vi "Main HMI.vi"() -> ()   [LabVIEW 2020]
uses:
  Control/State - Main HMI.ctl
  Control/Page List Configuration.ctl
  <vilib>/Utility/miscctls.llb/LVRectTypeDef.ctl
  Control/Setup - Sequence Data.ctl
  <vilib>/Utility/miscctls.llb/LVPointTypeDef.ctl
  <vilib>/Utility/miscctls.llb/LVPositionTypeDef.ctl
  Control/State - FGV.ctl
  <vilib>/picture/picture.llb/imagedata.ctl
  Control/Header - Page.ctl
  <vilib>/Utility/miscctls.llb/LVBoundsTypeDef.ctl
  Control/State - eFGV.ctl
  Control/Header - User Management.ctl
  Control/Section.ctl
  <vilib>/Platform/browser.llb/Open URL in Default Browser (string).vi
panel:
  out "Project Name":string
  out "Version":string="v1.0"
  in  "Developer":bool
  out "Logo":picture
  in  "Acquire":bool
  out "Log Time":dbl format="%<%H:%M:%S>t"
  in  "Log":bool
  in  "Left":bool caption="1"
  in  "Page":T1(radio)=enum."2"
  in  "Right":bool caption="11"
  in  "Screenshot":bool
  in  "Info":bool
  in  "Alarm Event":bool
  in  "Logout":bool
  in  "Close":bool
  out "Disable":bool
  in  "Error in":errorcluster
  out "Error out":errorcluster
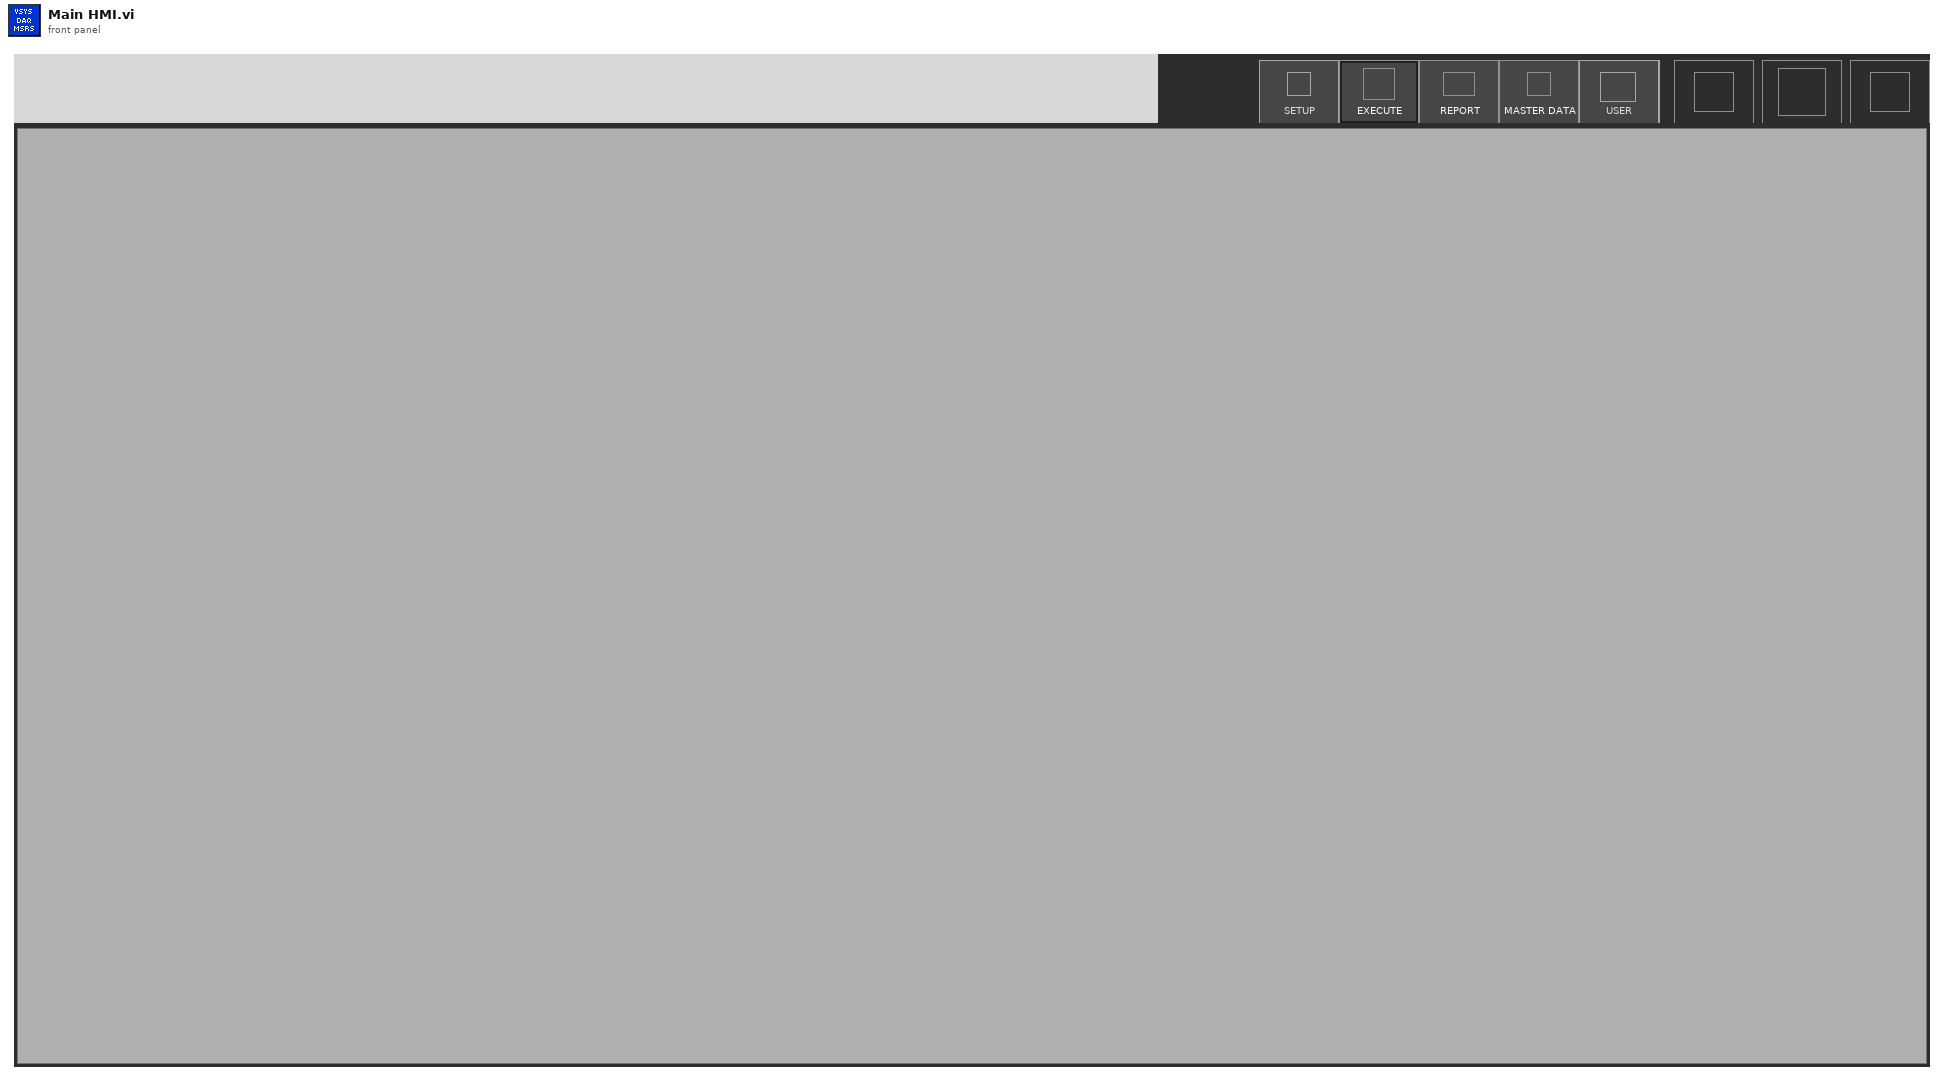
[diagram p1: front panel]
types:
  T1 = enum32{"1", "2", "3", "4", "5", "6", "7", "8", "9", "10", "11", "12", "13", "14", "15"}
  T2 = typedef "Page List Configuration.ctl" = cluster{"HMI Configuration":cluster{"EXE Name":string, "Project Name":string, "Max Page No":i32, "HMI State":enum32{"Invalid", "Standard", "Closed", "Hidden", "Minimized", "Maximized"}, "Version":enum16{"Demo", "User"}, "Check License":bool, "Font Size":u32, "Res: Height":i16, "Res: Width":i16, "License Level":enum16{"Level 1", "Level 2", "Level 3", "Level 4", "Level 5"}, "License Type":enum16{"Free", "Trial", "Subscription", "Perpetual"}}, "All HMI Module":string[], "Default HMI Module":string[], "Page Module":string[], "Page List: Level 1":string[], "Page List: Level 2":string[], "Page List: Level 3":string[], "All RT Module":string[], "Default RT Module":string[], "Acquire Enable Page":string[], "Log Enable Page":string[], "Run Page":string[], "Kill Page":string[], "Button":cluster{"Text":string[], "Tip Strip":string[]}}
  T3 = typedef "LVRectTypeDef.ctl" = cluster{"Left":i16, "Top":i16, "Right":i16, "Bottom":i16}
  T4 = typedef "Setup - Sequence Data.ctl" = cluster{"Seq.Select":bool, "Seq.Status":u32, "Seq.Run":bool, "Seq.TestSequence":string, "Seq.No":string, "Seq.ReqID":string, "Seq.TestReq":string, "Seq.Variance":string, "Seq.TestProcedure":string, "Seq.Section":string, "Seq.TestBunker":string, "Seq.TestMedia":string, "Seq.TestPressure":string, "Seq.Cycle":string, "Seq.HoldingTime":string, "Seq.ChartScale":string, "Seq.BDIndicator":string, "Seq.ActuatorPressure":string, "Seq.MaxBDPressure":string}
  T5 = cluster{"Config":T2, "Module":cluster{"Run Module":string[], "Kill Module":string[], "Page Module":string[], "Enable Page":string[]}, "Page Name":string, "T_Out":i32, "Time":timestamp, "Acquire":bool, "Log":bool, "Login":bool, "Discover":bool, "Button Ref":refnum<vi>[], "Direction":string, "Page Size":i32, "Content Area Rect":T3, "Page Size (Hidden)":i32, "Force Logout?":bool, "Update Button":bool, "Sequence Data":T4[], "Event Ref":refnum<event-registration>}
  T6 = typedef "State - Main HMI.ctl" = enum16{"Init", "Init Logo & Name", "Init Size", "Init Page", "Init Button Page", "Init Splitter", "Register Events", "Init Module", "Run Module", "Kill Module", "Change Page", "Update Button Page", "Close Splash Screen", "Idle", "Screenshot", "Developer Mode", "Info", "Move Button Page", "Acquire Event", "Log Event", "Logout", "Check for Exit", "Close"}
  T7 = enum32{"invalid app kind", "Development System", "Run Time System", "Student Edition", "Embedded LabVIEW", "Evaluation", "Custom"}
  T8 = typedef "LVPositionTypeDef.ctl" = cluster{"Left":i32, "Top":i32}
  T9 = typedef "State - FGV.ctl" = enum16{"Write", "Read"}
  T10 = typedef "imagedata.ctl" = cluster{"image type":i32, "image depth":i32, "image":u8[], "mask":u8[], "colors":u32[], "Rectangle":cluster{"left":i16, "top":i16, "right":i16, "bottom":i16}}
  T11 = enum16{"Init", "Init Module", "Run Module", "Kill Module", "Change Page", "Exit"}
  T12 = typedef "Header - Page.ctl" = enum16{"P1 Main", "P2", "P3 Analysis", "P4 Prediction", "P5 User"}
  T13 = enum8{"Enabled", "Disabled", "Disabled and Grayed Out"}
  T14 = typedef "LVBoundsTypeDef.ctl" = cluster{"Width":u32, "Height":u32}
  T15 = typedef "Header - User Management.ctl" = enum16{"Name", "Staff ID", "Username", "Password", "Access Level", "Status", "Access Page"}
  T16 = enum32{"Invalid", "Standard", "Closed", "Hidden", "Minimized", "Maximized"}
  T17 = typedef "Section.ctl" = enum16{"Software Setup", "Config", "Setup", "Network Stream", "MQTT Client", "Setting", "Sample Interval", "Calibration", "Pre-Ranging", "Overrun", "Static", "Filter", "Properties", "Alarm", "Device", "Logging"}
  T18 = typedef "LVPointTypeDef.ctl" = cluster{"Horizontal":i16, "Vertical":i16}
  T19 = typedef "State - eFGV.ctl" = enum16{"Init", "Read", "Write", "Exit"}
  T20 = typedef "License File Parameter.ctl" = cluster{"Expired Time":string, "Computer ID":string, "Product Name":string, "Period":i16, "Activated Time":string, "License Level":enum16{"Level 1", "Level 2", "Level 3", "Level 4", "Level 5"}, "License Type":enum16{"Free", "Trial", "Subscription", "Perpetual"}, "Log Time":string}
  T21 = enum16{"Free", "Trial", "Subscription", "Perpetual"}
  T22 = cluster{"Page Name":string, "All Module":string[], "Default Run Module":string[], "Page Module":string[]}
  T23 = enum16{"Level 1", "Level 2", "Level 3", "Level 4", "Level 5"}
  T24 = enum16{"Pre-Ranging", "Overrun", "Static", "Analysis", "Prediction"}
  T25 = enum32{"Bad", "Idle", "Run top level", "Running"}
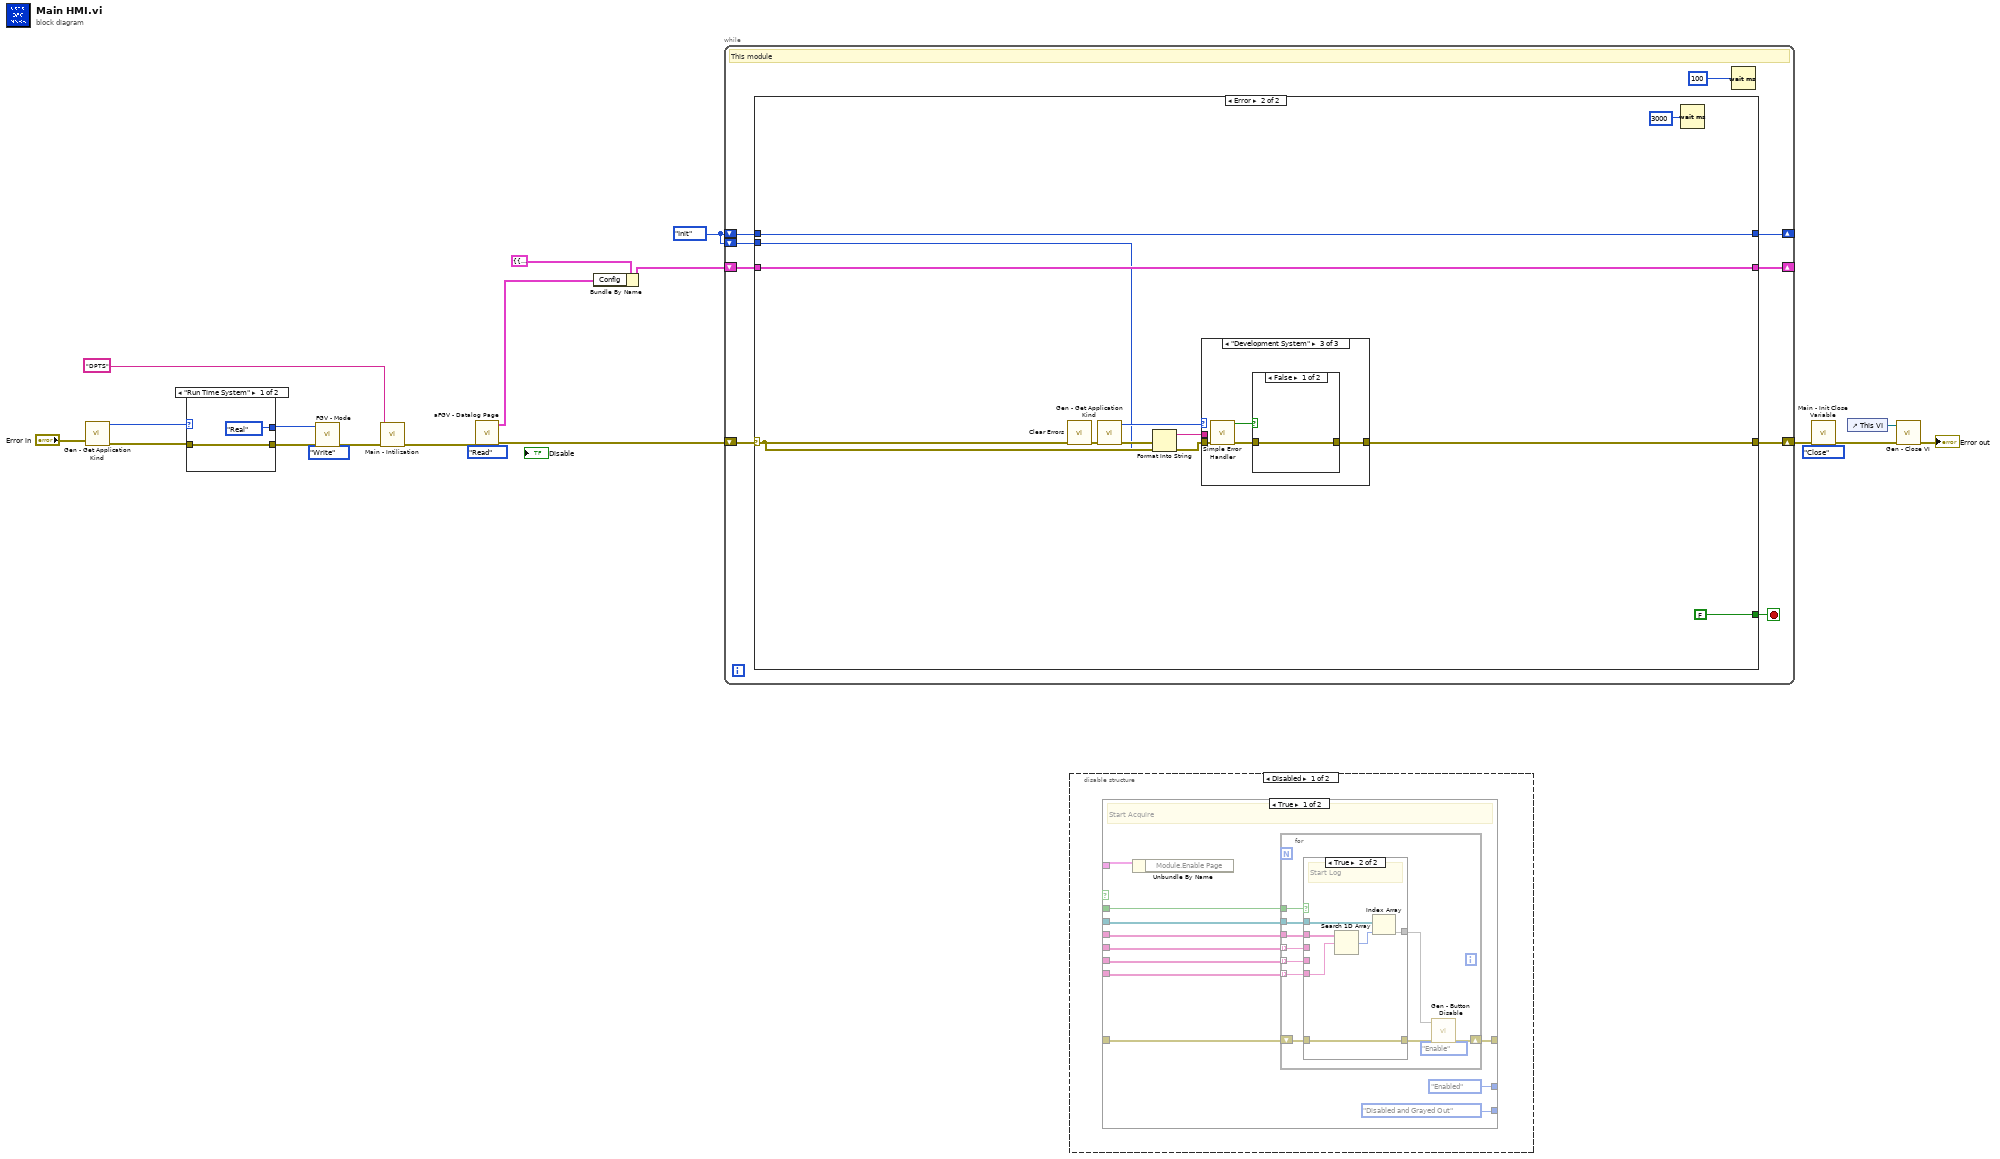
[diagram p0: block diagram]
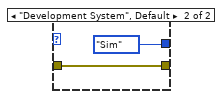
[diagram p2: hidden frame]
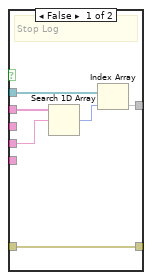
[diagram p3: hidden frame]
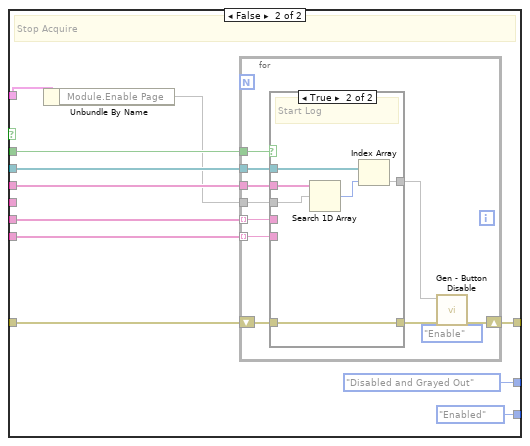
[diagram p4: hidden frame]
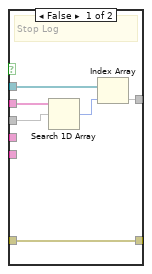
[diagram p5: hidden frame]
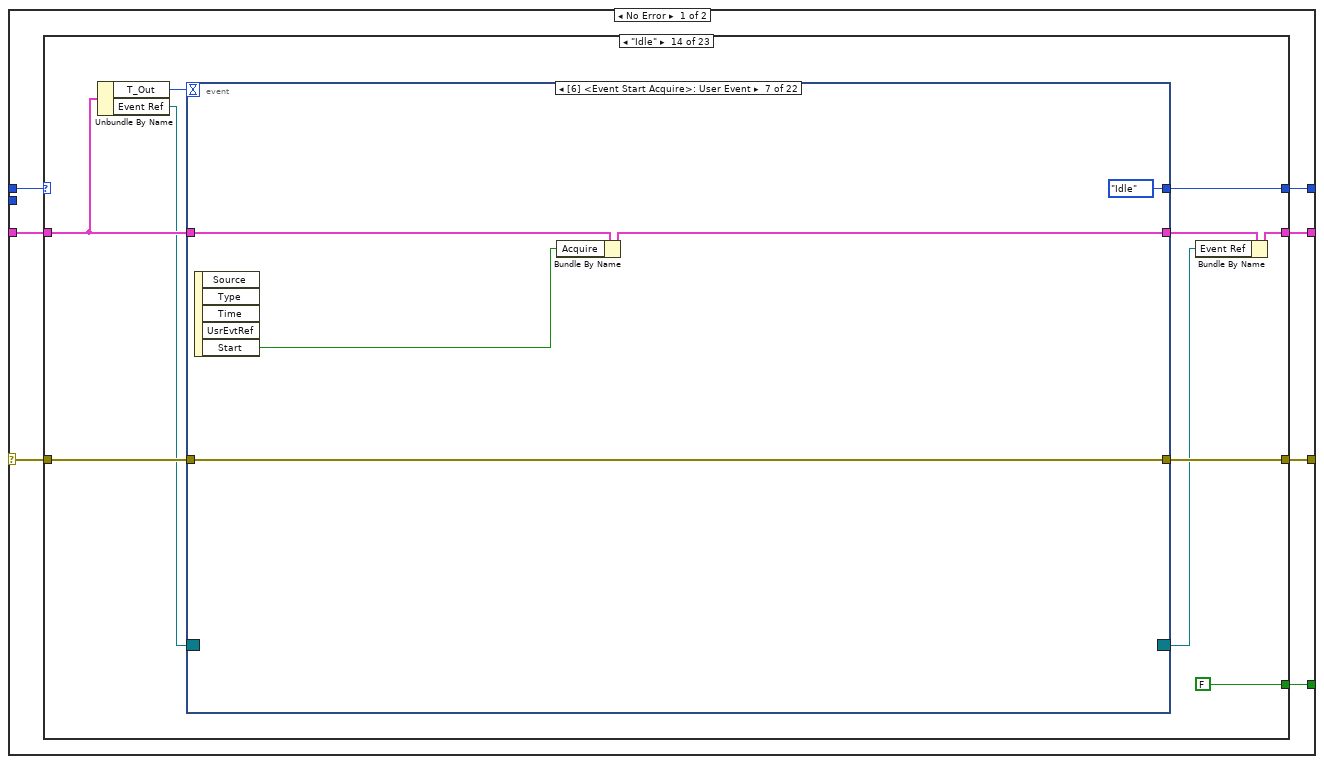
[diagram p7: hidden frame]
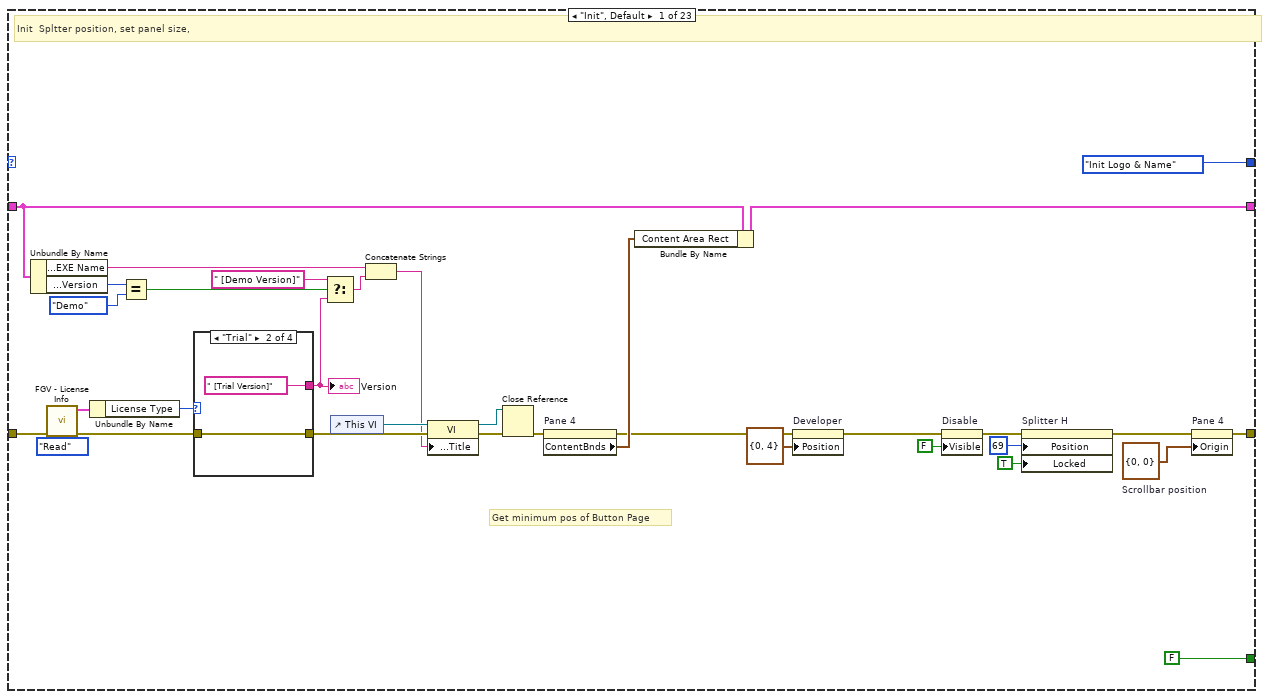
[diagram p8: hidden frame]
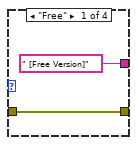
[diagram p9: hidden frame]
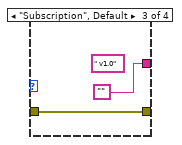
[diagram p10: hidden frame]
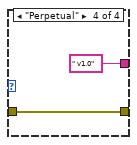
[diagram p11: hidden frame]
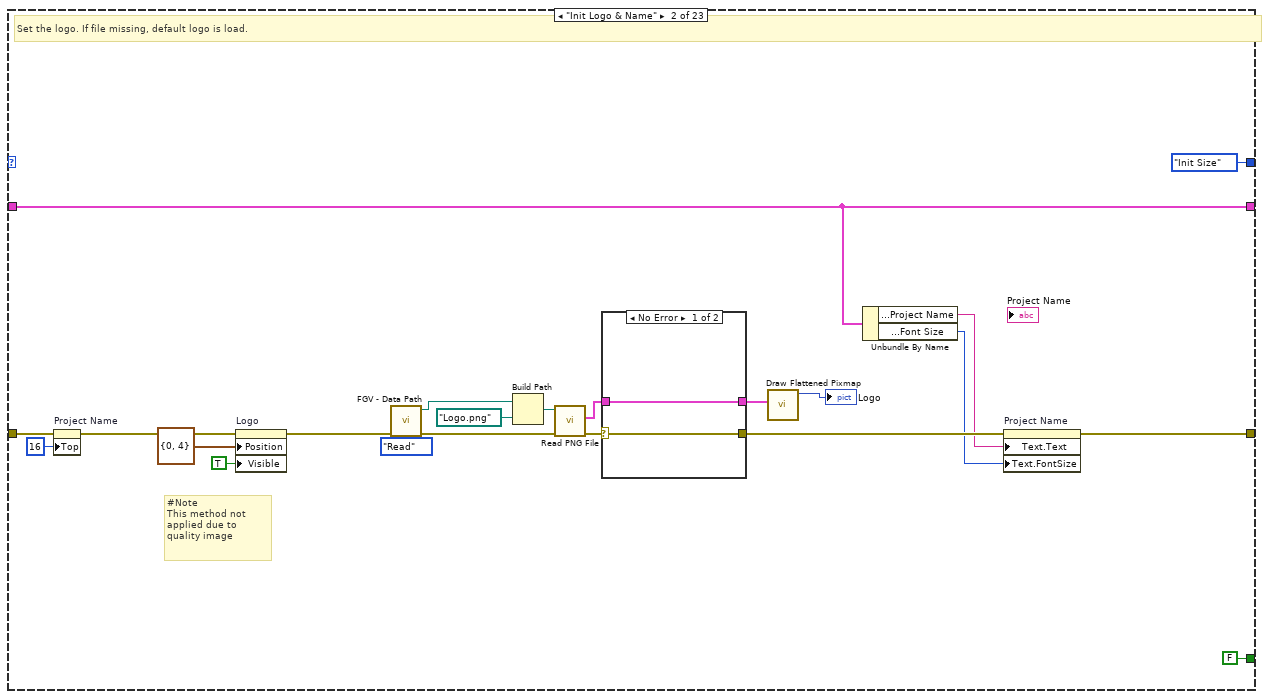
[diagram p12: hidden frame]
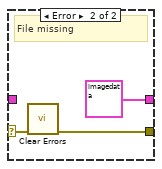
[diagram p13: hidden frame]
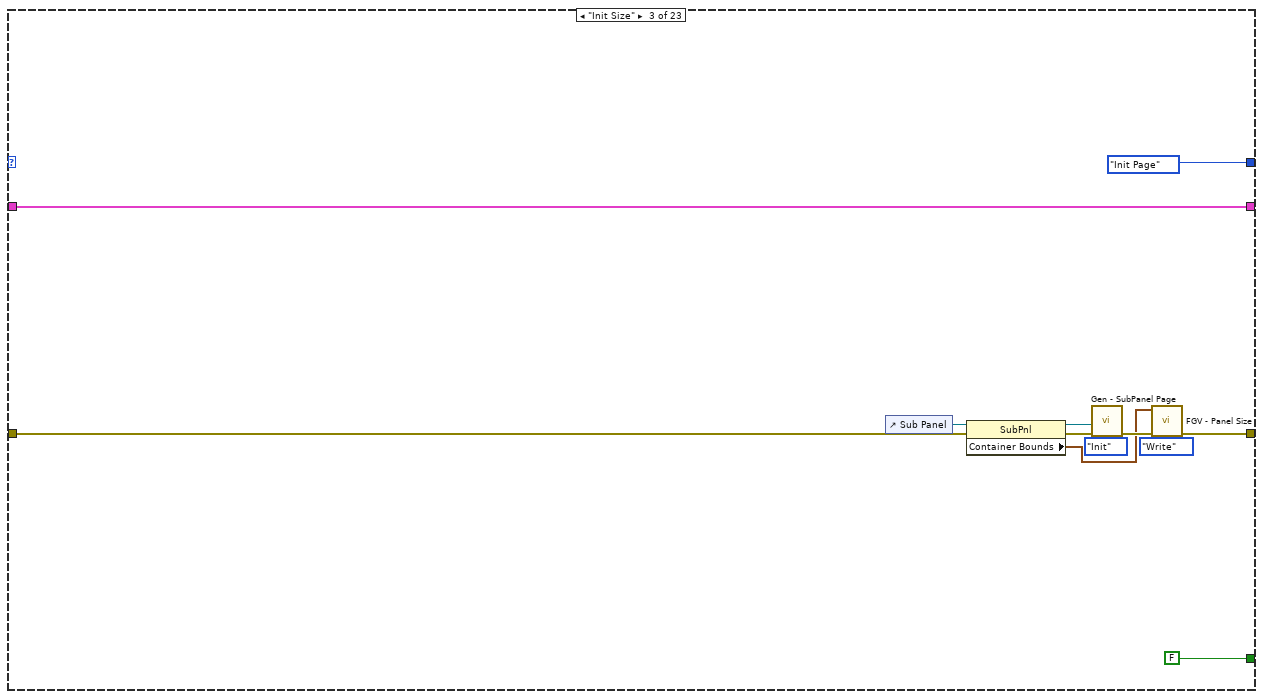
[diagram p14: hidden frame]
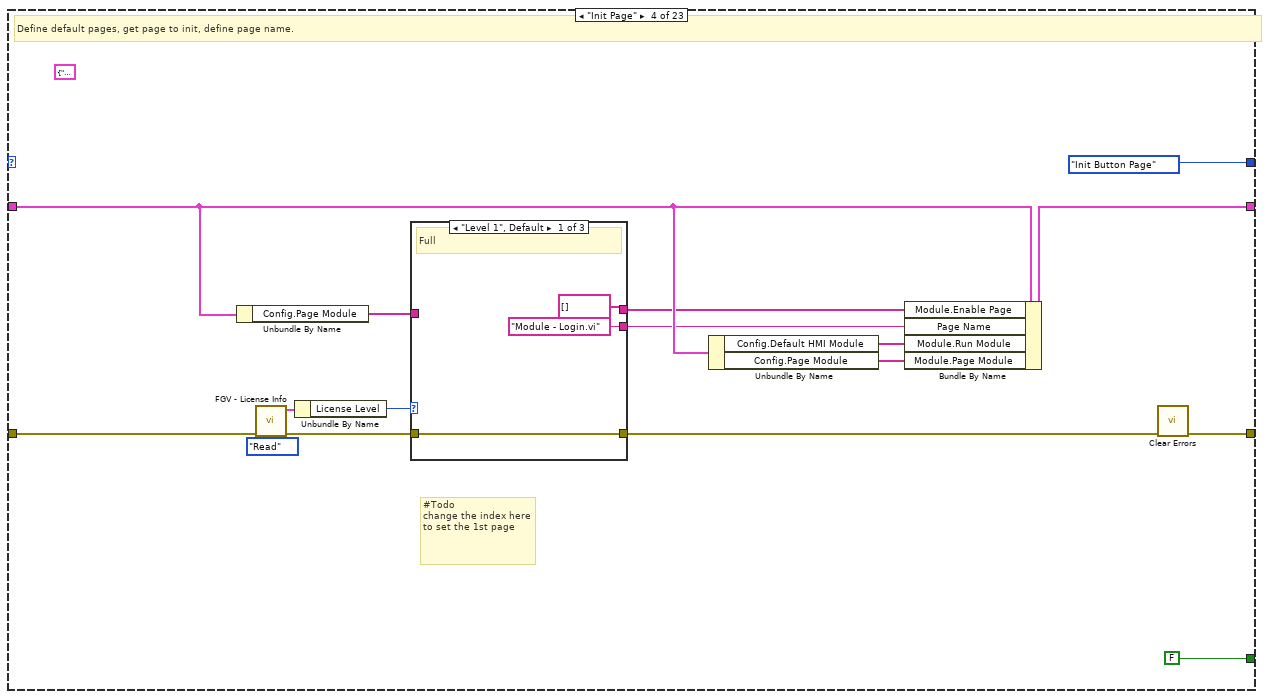
[diagram p15: hidden frame]
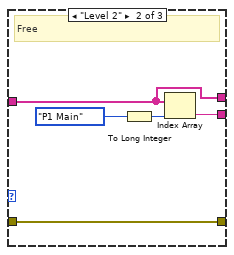
[diagram p16: hidden frame]
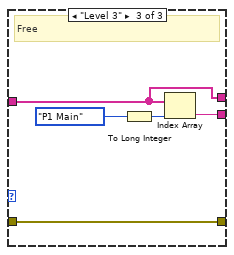
[diagram p17: hidden frame]
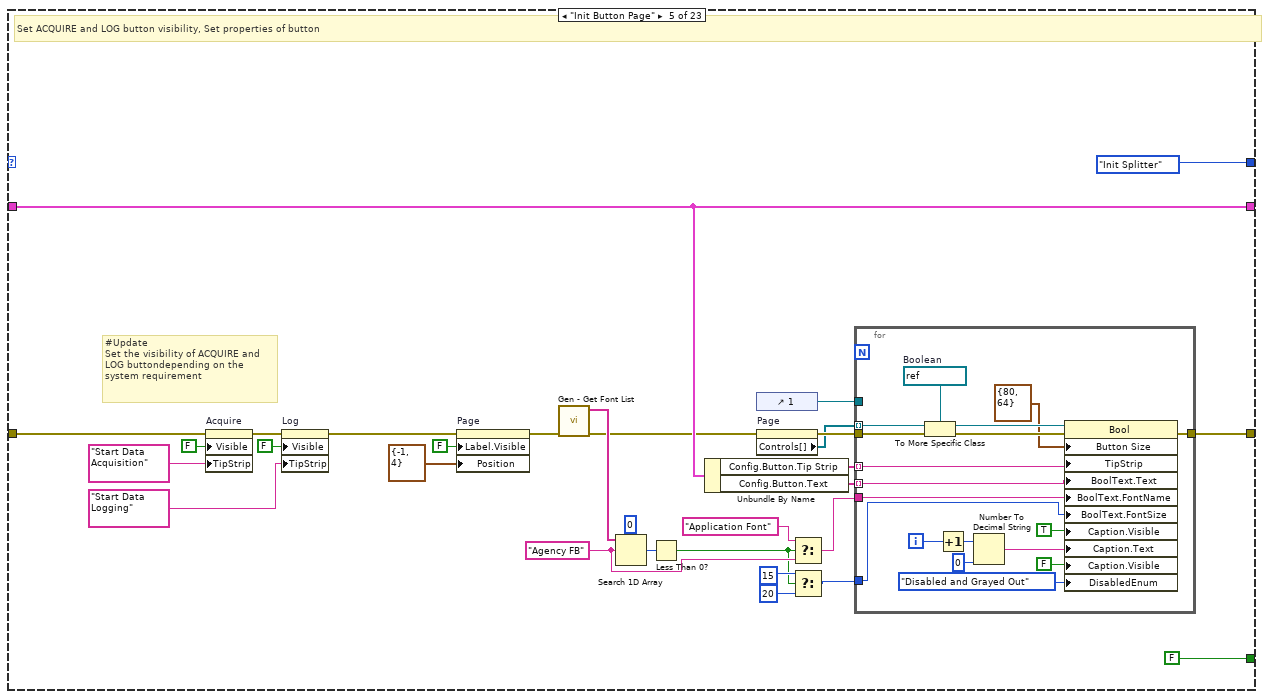
[diagram p18: hidden frame]
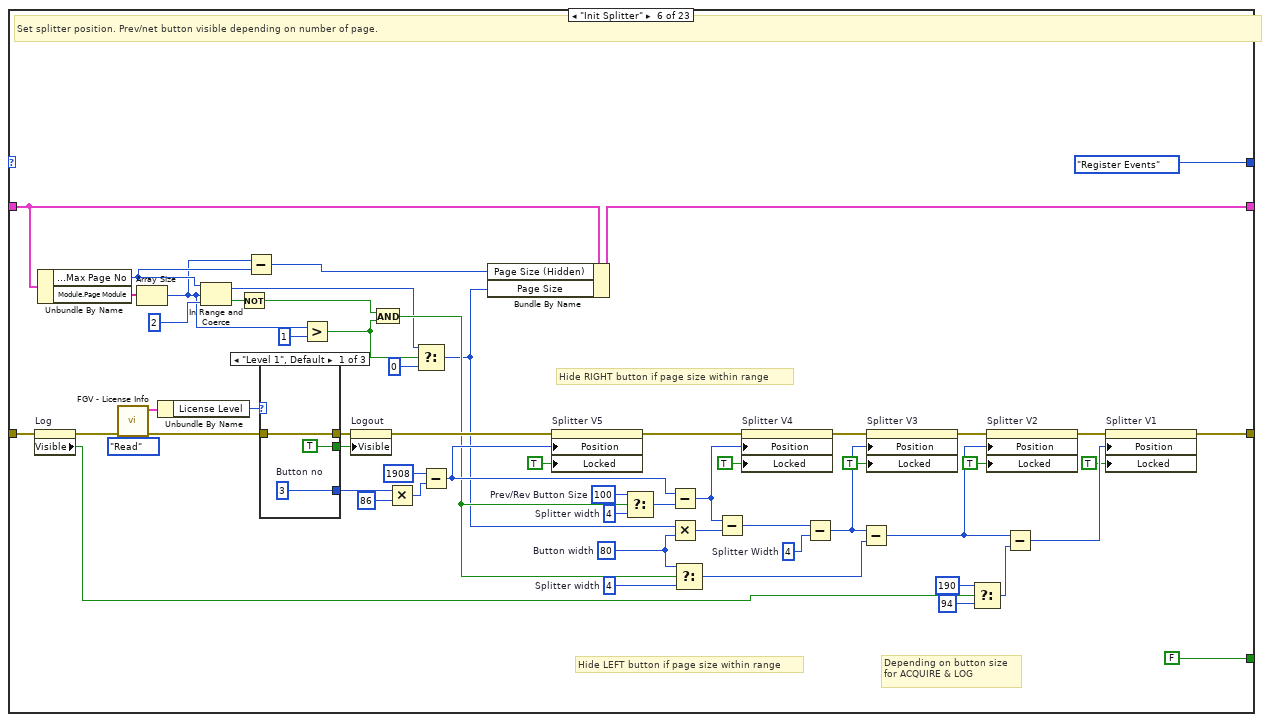
[diagram p19: hidden frame]
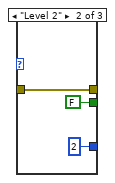
[diagram p20: hidden frame]
diagram:
  w14 = State_-_Main_HMI."Init"
  n1 = call "Gen - Get Application Kind.vi"("Error In"="Error in") -> ("Error Out"=w9:errorcluster, "Application:Kind"=w8:T7)  [unwired: 9 in]
  n2 = case shown="\"Run Time System\"" w8 {
    tunnel: [enum16{"Sim", "Real"}."Real" ("Mode in") enum16{"Sim", "Real"}."Sim" ("Mode in")] -> w5
    tunnel: w9 -> [w21 w23]
    tunnel: [w21 w23] -> w6
    frame "Run Time System" {
    }
    frame "Development System", Default {
    }
  }
  n3 = call "FGV - Mode.vi"("Action"=enum16{"Read", "Write"}."Write", "Error In"=w6, "Mode in"=w5) -> ("Error Out"=w4:errorcluster)  [unwired: 7 in, 1 out]
  n4 = call "Main - Intilization.vi"("Error In"=w4, "Exe Name"="DPTS") -> ("Error Out"=w3:errorcluster)  [unwired: 9 in]
  n5 = call "aFGV - Datalog Page.vi"("Action"=enum16{"Read", "Write"}."Read", "Error In"=w3) -> ("Error Out"=w1:errorcluster, "Data Out"=w11:T2)  [unwired: 8 in]
  n6 = Bundle By Name(cluster=T5 {"Config"={"HMI Configuration"={"EXE Name"="", "Project Name"="", "Max Page No"=2, "HMI State"=enum."Maximized", "Version"=enum."Demo", "Check License"=FALSE, "Font Size"=44, "Res: Height"=655, "Res: Width"=1356, "License Level"=enum."Level 2", "License Type"=enum."Perpetual"}, "All HMI Module"=["Module - DAQmx AI Daemon.vit", "Module - DAQmx AI.vi", "Module - DAQmx AO.vi", "Module - DAQmx DI.vi", "Module - DAQmx DO.vi", "Module - Error Management.vi", "Module - Login.vi", "Module - P1 Display.vi", "Module - P2 List Device.vi", "Module - P3 Configure Tags IO.vi", "Module - P4 Log Config.vi", "Module - P5 Filter.vi", "Module - P6 Calibration.vi", "Module - P7 Analysis.vi", "Module - P8 User Management.vi"], "Default HMI Module"=["Module - Error Management.vi", "Module - Login.vi", "Module - P1 Display.vi", "Module - P2 List Device.vi", "Module - P3 Configure Tags IO.vi", "Module - P4 Log Config.vi", "Module - P5 Filter.vi", "Module - P6 Calibration.vi", "Module - P7 Analysis.vi", "Module - P8 User Management.vi"], "Page Module"=["Module - P1 Display.vi", "Module - P2 List Device.vi", "Module - P3 Configure Tags IO.vi", "Module - P4 Log Config.vi", "Module - P5 Filter.vi", "Module - P6 Calibration.vi", "Module - P7 Analysis.vi", "Module - P8 User Management.vi"], "Page List: Level 1"=[], "Page List: Level 2"=[], "Page List: Level 3"=[], "All RT Module"=[], "Default RT Module"=[], "Acquire Enable Page"=[], "Log Enable Page"=[], "Run Page"=[], "Kill Page"=[], "Button"={"Text"=["", "", "", "", "", "", "", ""], "Tip Strip"=[]}}, "Module"={"Run Module"=[], "Kill Module"=[], "Page Module"=[], "Enable Page"=[]}, "Page Name"="", "T_Out"=-1, "Time"=timestamp(0 s since 1904-01-01), "Acquire"=FALSE, "Log"=FALSE, "Login"=FALSE, "Discover"=FALSE, "Button Ref"=[], "Direction"="", "Page Size"=0, "Content Area Rect"={"Left"=0, "Top"=0, "Right"=0, "Bottom"=0}, "Page Size (Hidden)"=0, "Force Logout?"=FALSE, "Update Button"=TRUE, "Sequence Data"=[], "Event Ref"=refnum}, "Config"=w11) -> (w12:T5)
  n7 = while {
    shift-right: [w29] -> _
    shift-left: w14 -> [w32]
    shift-right: [w31] -> w18
    shift-left: w1 -> [w33]
    shift-right: [w27] -> _
    shift-left: w12 -> [w28]
    shift-left: w14 -> [w25]
    stop <- w30 stop-if-true
    # "This module"
    n8 = case shown="Error" w33 {
      selector: w33 -> [w38 w1037]
      tunnel: w32 -> [w40 w1042]
      tunnel: [w39 w1036] -> w31
      tunnel: [w37 FALSE] -> w30
      tunnel: [w36 w1042] -> w29
      tunnel: w28 -> [w35 w1041]
      tunnel: [w34 w1041] -> w27
      tunnel: w25 -> [_ w1034]
      frame No Error {
        n9 = case shown="\"Idle\"" w40 {
          tunnel: [w65 w84 w110 w128 w176 w248 w303 w315 w322 w329 w357 w384 w506 w518 w704 w733 w781 w794 w833 w862 w918 w960 w1004] -> w39
          tunnel: w38 -> [w64 w88 w109 w127 w151 w213 w269 w313 w321 w328 w350 w387 w507 w517 w724 w737 w779 w792 w838 w867 w916 w963 w1005]
          tunnel: [FALSE FALSE FALSE FALSE FALSE FALSE FALSE FALSE FALSE FALSE FALSE FALSE FALSE FALSE FALSE FALSE FALSE FALSE FALSE FALSE FALSE FALSE TRUE] -> w37
          tunnel: [State_-_Main_HMI."Init Logo & Name" State_-_Main_HMI."Init Size" State_-_Main_HMI."Init Page" State_-_Main_HMI."Init Button Page" State_-_Main_HMI."Init Splitter" State_-_Main_HMI."Register Events" State_-_Main_HMI."Init Module" State_-_Main_HMI."Run Module" State_-_Main_HMI."Kill Module" State_-_Main_HMI."Change Page" w335 w388 State_-_Main_HMI."Idle" w515 State_-_Main_HMI."Idle" State_-_Main_HMI."Idle" State_-_Main_HMI."Idle" State_-_Main_HMI."Idle" w827 State_-_Main_HMI."Update Button Page" w922 w966 State_-_Main_HMI."Close"] -> w36
          tunnel: w35 -> [w46 w89 w120 w126 w173 w241 w307 w309 w319 w326 w353 w375 w498 w513 w730 w738 w783 w804 w837 w866 w919 w968 w986]
          tunnel: [w71 w89 w120 w134 w173 w232 w272 w309 w319 w326 w340 w375 w498 w510 w730 w738 w783 w804 w826 w864 w920 w968 w986] -> w34
          frame "Init", Default {
            w67 = T18 {"Horizontal"=0, "Vertical"=0}  # Scrollbar position
            # "Get minimum pos of Button Page"
            # "Init  Spltter position, set panel size,"
            n10 = Unbundle By Name(w46) -> ("Config.HMI Configuration.EXE Name"=w44:string, "Config.HMI Configuration.Version"=w45:enum16{"Demo", "User"})
            n11 = call "FGV - License Info.vi"("FGV States"=enum16{"Read", "Write"}."Read", "Error In"=w64) -> ("Error Out"=w60:errorcluster, "License Info"=w62:T20)  [unwired: 8 in]
            n12 = Unbundle By Name(w62) -> ("License Type"=w61:T21)
            n13 = Equal?(x=w45, y=enum16{"Demo", "User"}."Demo") -> (x = y?=w53:bool)
            n14 = case shown="\"Trial\"" w61 {
              tunnel: [w74 w76 w79 w80] -> w55
              tunnel: w60 -> [w74 w76 w79 w80]
              tunnel: [" [Free Version]" ("Version") " [Trial Version]" ("Version") "" " v1.0" ("Version")] -> w52
              frame "Free" {
              }
              frame "Trial" {
              }
              frame "Subscription", Default {
                (unwired) " v1.0" ("Version")
              }
              frame "Perpetual" {
              }
            }
            "Version" <- w52
            n15 = Select(t=" [Demo Version]", s=w53, f=w52) -> (s? t:f=w51:string)
            n16 = control-ref of="This VI"() -> (w59:refnum<vi>)
            n17 = Concatenate Strings(w44, w51) -> (w49:string)
            n18 = property class="VI"(reference=w59, error in=w55, "Front Panel.Title"=w49) -> (reference out=w58:refnum<vi>, error out=w57:errorcluster)
            n19 = Close Reference(reference=w58, error in (no error)=w57) -> (error out=w56:errorcluster)
            n20 = property on="Pane 4" class="Pane"(error in=w56) -> (error out=w43:errorcluster, "ContentBnds"=w70:T3)  [unwired: 1 in, 1 out]
            n21 = Bundle By Name(cluster=w46, "Content Area Rect"=w70) -> (w71:T5)
            n22 = property on="Developer" class="Bool (strict)"(error in=w43, "Position"=T8 {"Left"=0, "Top"=4}) -> (error out=w42:errorcluster)  [unwired: 1 in, 1 out]
            n23 = property on="Disable" class="Bool (strict)"(error in=w42, "Visible"=FALSE) -> (error out=w48:errorcluster)  [unwired: 1 in, 1 out]
            n24 = property on="Splitter H" class="Splitter"(error in=w48, "Position"=69 ("Splitter Position"), "Locked"=TRUE ("Splitter Position Locked")) -> (error out=w66:errorcluster)  [unwired: 1 in, 1 out]
            n25 = property on="Pane 4" class="Pane"(error in=w66, "Origin"=w67) -> (error out=w65:errorcluster)  [unwired: 1 in, 1 out]
          }
          frame "Init Logo & Name" {
            # "#Note\nThis method not applied due to quality image"
            # "Set the logo. If file missing, default logo is load."
            n26 = property on="Project Name" class="Str"(error in=w88, "Top"=16 ("Position:Top")) -> (error out=w87:errorcluster)  [unwired: 1 in, 1 out]
            n27 = property on="Logo" class="Pict"(error in=w87, "Position"=T8 {"Left"=0, "Top"=4}, "Visible"=TRUE) -> (error out=w93:errorcluster)  [unwired: 1 in, 1 out]
            n28 = call "FGV - Data Path.vi"("FGV State"=State_-_FGV."Read", "Error In"=w93) -> ("Error Out"=w96:errorcluster, "Path Out"=w97:path)  [unwired: 8 in]
            n29 = Build Path(base path=w97, name or relative path=path "Logo.png") -> (appended path=w101:path)
            n30 = call <vilib>:"Read PNG File.vi"("error in (no error)"=w96, "path to PNG file"=w101) -> ("error out"=w99:errorcluster, "image data"=w98:T10)  [unwired: 7 in, 1 out]
            n31 = case shown="No Error" w99 {
              selector: w99 -> [w105 w108]
              tunnel: [w105 w106] -> w85
              tunnel: [w104 T10 {"image type"=0, "image depth"=32, "image"=array[57088 elements], "mask"=array[1792 elements], "colors"=[], "Rectangle"={"left"=0, "top"=0, "right"=223, "bottom"=64}} ("image data")] -> w91
              tunnel: w98 -> [w104 _]
              frame No Error {
              }
              frame Error {
                # "File missing"
                n32 = call <vilib>:"Clear Errors.vi"("error in (no error)"=w108) -> ("error out"=w106:errorcluster)  [unwired: 5 in, 1 out]
              }
            }
            n33 = call <vilib>:"Draw Flattened Pixmap.vi"("image data"=w91) -> ("new picture"=→"Logo":picture)  [unwired: 8 in]
            n34 = Unbundle By Name(w89) -> ("Config.HMI Configuration.Project Name"=w83:string, "Config.HMI Configuration.Font Size"=w82:u32)
            n35 = property on="Project Name" class="Str"(error in=w85, "Text.Text"=w83, "Text.FontSize"=w82) -> (error out=w84:errorcluster)  [unwired: 1 in, 1 out]
          }
          frame "Init Size" {
            n36 = control-ref of="Sub Panel"() -> (w117:refnum<vi>)
            n37 = property class="SubPnl"(reference=w117, error in=w109) -> (reference out=w115:refnum<vi>, error out=w116:errorcluster, "Container Bounds"=w113:T14)
            n38 = call "Gen - SubPanel Page.vi"("State"=T11."Init", "Error In"=w116, "Main SubPanel Ref"=w115) -> ("Error Out"=w114:errorcluster)  [unwired: 8 in]
            n39 = call "FGV - Panel Size.vi"("Action"=enum16{"Read", "Write"}."Write", "Error In"=w114, "Size In"=w113) -> ("Error Out"=w110:errorcluster)  [unwired: 7 in, 1 out]
          }
          frame "Init Page" {
            (unwired) T22 {"Page Name"="Module - Login.vi", "All Module"=["Module - DAQmx AI Daemon.vit", "Module - DAQmx AI.vi", "Module - DAQmx AO.vi", "Module - DAQmx DI.vi", "Module - DAQmx DO.vi", "Module - Data Log.vi", "Module - Error Management.vi", "Module - Login.vi", "Module - P1 Display.vi", "Module - P2 List Device.vi", "Module - P3 Configure Tags IO.vi", "Module - P4 Log Config.vi", "Module - P5 Filter.vi", "Module - P6 Calibration.vi", "Module - P7 Analysis.vi", "Module - P8 User Management.vi"], "Default Run Module"=["Module - Error Management.vi", "Module - Login.vi", "Module - P1 Display.vi", "Module - P2 List Device.vi", "Module - P3 Configure Tags IO.vi", "Module - P4 Log Config.vi", "Module - P5 Filter.vi", "Module - P6 Calibration.vi", "Module - P7 Analysis.vi", "Module - P8 User Management.vi"], "Page Module"=["Module - P1 Display.vi", "Module - P2 List Device.vi", "Module - P3 Configure Tags IO.vi", "Module - P4 Log Config.vi", "Module - P5 Filter.vi", "Module - P6 Calibration.vi", "Module - P7 Analysis.vi", "Module - P8 User Management.vi"]}
            # "#Todo \nchange the index here to set the 1st page"
            # "Define default pages, get page to init, define page name."
            n40 = Unbundle By Name(w126) -> ("Config.Page Module"=w124:string[])
            n41 = call "FGV - License Info.vi"("FGV States"=enum16{"Read", "Write"}."Read", "Error In"=w127) -> ("Error Out"=w130:errorcluster, "License Info"=w132:T20)  [unwired: 8 in]
            n42 = Unbundle By Name(w132) -> ("License Level"=w129:T23)
            n43 = case shown="\"Level 1\", Default" w129 {
              tunnel: [w139 w144 w149] -> w131
              tunnel: w130 -> [w139 w144 w149]
              tunnel: w124 -> [_ w140 w145]
              tunnel: ["Module - Login.vi" ("String") w142 w147] -> w123
              tunnel: [string[] [] ("Page Module") w140 w145] -> w122
              frame "Level 1", Default {
                # "Full"
              }
              frame "Level 2" {
                # "Free"
                n44 = To Long Integer(number=Header_-_Page."P1 Main" ("Header - Page")) -> (32bit integer=w141:i32)
                n45 = Index Array(array=w140, index=w141) -> (element=w142:string)
              }
              frame "Level 3" {
                # "Free"
                n46 = To Long Integer(number=Header_-_Page."P1 Main" ("Header - Page")) -> (32bit integer=w146:i32)
                n47 = Index Array(array=w145, index=w146) -> (element=w147:string)
              }
            }
            n48 = Unbundle By Name(w126) -> ("Config.Default HMI Module"=w125:string[], "Config.Page Module"=w121:string[])
            n49 = Bundle By Name(cluster=w126, "Module.Enable Page"=w122, "Page Name"=w123, "Module.Run Module"=w125, "Module.Page Module"=w121) -> (w134:T5)
            n50 = call <vilib>:"Clear Errors.vi"("error in (no error)"=w131) -> ("error out"=w128:errorcluster)  [unwired: 5 in, 1 out]
          }
          frame "Init Button Page" {
            (unwired) 0 ("y")
            w168 = "Agency FB" ("Boolean Text.Font:Name")
            # "#Update\nSet the visibility of ACQUIRE and LOG buttondepending on the system requirement"
            # "Set ACQUIRE and LOG button visibility, Set properties of button"
            n51 = property on="Acquire" class="Bool (strict)"(error in=w151, "Visible"=FALSE, "TipStrip"="Start Data Acquisition" ("Tip Strip")) -> (error out=w156:errorcluster)  [unwired: 1 in, 1 out]
            n52 = property on="Log" class="Bool (strict)"(error in=w156, "Visible"=FALSE, "TipStrip"="Start Data Logging" ("Tip Strip")) -> (error out=w150:errorcluster)  [unwired: 1 in, 1 out]
            n53 = property on="Page" class="RadioBtnsControl (strict)"(error in=w150, "Label.Visible"=FALSE, "Position"=T8 {"Left"=-1, "Top"=4}) -> (error out=w158:errorcluster)  [unwired: 1 in, 1 out]
            n54 = call "Gen - Get Font List.vi"("Error In"=w158) -> ("Error Out"=w161:errorcluster, "Font List"=w162:string[])  [unwired: 9 in]
            n55 = Search 1D Array(1D array=w162, element=w168) -> (index of element=w170:i32)  [unwired: 1 in]
            n56 = Less Than 0?(x=w170) -> (x < 0?=w164:bool)
            n57 = Unbundle By Name(w173) -> ("Config.Button.Tip Strip"=w157:string[], "Config.Button.Text"=w172:string[])
            n58 = control-ref of="1"() -> (w174:refnum<vi>)
            n59 = property on="Page" class="RadioBtnsControl (strict)"(error in=w161) -> (error out=w175:errorcluster, "Controls[]"=w171:refnum<vi>[])  [unwired: 1 in, 1 out]
            n60 = Select(t="Application Font" ("Boolean Text.Font:Name"), s=w164, f=w168) -> (s? t:f=w167:string)
            n61 = Select(t=u32 15 ("Boolean Text.Font:Size"), s=w164, f=u32 20) -> (s? t:f=w165:u32)
            n62 = for {
              tunnel: [w196] -> w176
              tunnel: w175 -> [w189]
              tunnel: w171 -> [w191] mode=indexing
              tunnel: w174 -> [_]
              tunnel: w172 -> [w180] mode=indexing
              tunnel: w167 -> [w183]
              tunnel: w165 -> [w182]
              tunnel: w157 -> [w179] mode=indexing
              i -> [w194]
              w181 = refnum<vi> refnum  # Boolean
              n63 = To More Specific Class(target class=w181, reference=w191, error in=w189) -> (specific class reference=w192:refnum<vi>, error out=w190:errorcluster)
              n64 = Increment(x=w194) -> (x+1=w195:i32)
              n65 = Number To Decimal String(number=w195, width (-)=i16 0) -> (decimal integer string=w188:string)
              n66 = property class="Bool"(reference=w192, error in=w190, "Button Size"=T14 {"Width"=80, "Height"=64}, "TipStrip"=w179, "BoolText.Text"=w180, "BoolText.FontName"=w183, "BoolText.FontSize"=w182, "Caption.Visible"=TRUE, "Caption.Text"=w188, "Caption.Visible"=FALSE, "DisabledEnum"=T13."Disabled and Grayed Out" ("Disabled")) -> (error out=w196:errorcluster)  [unwired: 1 out]
            }
          }
          frame "Init Splitter" {
            w231 = 80  # Button width
            w234 = 4  # Splitter width
            w237 = 4  # Splitter width
            w239 = 100  # Prev/Rev Button Size
            w243 = 4  # Splitter Width
            # "Depending on button size for ACQUIRE & LOG"
            # "Hide LEFT button if page size within range"
            # "Hide RIGHT button if page size within range"
            # "Set splitter position. Prev/net button visible depending on number of page."
            n67 = property on="Log" class="Bool (strict)"(error in=w213) -> (error out=w212:errorcluster, "Visible"=w211:bool)  [unwired: 1 in, 1 out]
            n68 = Unbundle By Name(w241) -> ("Config.HMI Configuration.Max Page No"=w206:i32, "Module.Page Module"=w240:string[])
            n69 = call "FGV - License Info.vi"("FGV States"=enum16{"Read", "Write"}."Read", "Error In"=w212) -> ("Error Out"=w229:errorcluster, "License Info"=w228:T20)  [unwired: 8 in]
            n70 = Array Size(array=w240) -> (size(s)=w204:i32)
            n71 = Unbundle By Name(w228) -> ("License Level"=w230:T23)
            n72 = In Range and Coerce(upper limit=w206, x=w204, lower limit=2 ("HMI Configuration.Max Page No")) -> (coerced(x)=w198:i32, In Range?=w235:bool)
            n73 = Not(x=w235) -> (.not. x?=w202:bool)
            n74 = Subtract(x=w204, y=w206) -> (x-y=w205:i32)
            n75 = case shown="\"Level 1\", Default" w230 {
              tunnel: [w257 w260 w263] -> w225
              tunnel: w229 -> [w257 w260 w263]
              tunnel: [TRUE ("Visible") FALSE ("Visible") FALSE ("Visible")] -> w224
              tunnel: [w255 2 ("Button no") 2 ("Button no")] -> w214
              frame "Level 1", Default {
                w255 = 3  # Button no
              }
              frame "Level 2" {
              }
              frame "Level 3" {
              }
            }
            n76 = Greater?(x=w204, y=1) -> (0:w200:bool)
            n77 = property on="Logout" class="Bool"(error in=w225, "Visible"=w224) -> (error out=w226:errorcluster)  [unwired: 1 in, 1 out]
            n78 = And(x=w202, y=w200) -> (x .and. y?=w201:bool)
            n79 = Multiply(x=w214, y=86) -> (x*y=w215:i32)
            n80 = Select(t=w198, s=w200, f=0) -> (s? t:f=w197:i32)
            n81 = Subtract(x=1908 ("Splitter Position"), y=w215) -> (x-y=w216:i32)
            n82 = Bundle By Name(cluster=w241, "Page Size (Hidden)"=w205, "Page Size"=w197) -> (w232:T5)
            n83 = property on="Splitter V5" class="Splitter"(error in=w226, "Position"=w216, "Locked"=TRUE ("Splitter Position Locked")) -> (error out=w242:errorcluster)  [unwired: 1 in, 1 out]
            n84 = Select(t=w239, s=w201, f=w237) -> (s? t:f=w238:i32)
            n85 = Subtract(x=w216, y=w238) -> (x-y=w236:i32)
            n86 = Multiply(x=w197, y=w231) -> (x*y=w250:i32)
            n87 = Select(t=w231, s=w201, f=w234) -> (s? t:f=w233:i32)
            n88 = Subtract(x=w236, y=w250) -> (x-y=w245:i32)
            n89 = property on="Splitter V4" class="Splitter"(error in=w242, "Position"=w236, "Locked"=TRUE ("Splitter Position Locked")) -> (error out=w251:errorcluster)  [unwired: 1 in, 1 out]
            n90 = Subtract(x=w245, y=w243) -> (x-y=w244:i32)
            n91 = Subtract(x=w244, y=w233) -> (x-y=w247:i32)
            n92 = property on="Splitter V3" class="Splitter"(error in=w251, "Position"=w244, "Locked"=TRUE ("Splitter Position Locked")) -> (error out=w252:errorcluster)  [unwired: 1 in, 1 out]
            n93 = Select(t=190 ("y"), s=w211, f=94 ("y")) -> (s? t:f=w209:i32)
            n94 = property on="Splitter V2" class="Splitter"(error in=w252, "Position"=w247, "Locked"=TRUE ("Splitter Position Locked")) -> (error out=w249:errorcluster)  [unwired: 1 in, 1 out]
            n95 = Subtract(x=w247, y=w209) -> (x-y=w246:i32)
            n96 = property on="Splitter V1" class="Splitter"(error in=w249, "Position"=w246, "Locked"=TRUE ("Splitter Position Locked")) -> (error out=w248:errorcluster)  [unwired: 1 in, 1 out]
          }
          frame "Register Events" {
            w267 = State_-_eFGV."Read" ("FGV State")
            # "Register related events."
            n97 = control-ref of="1"() -> (w299:refnum<vi>)
            n98 = control-ref of="2"() -> (w298:refnum<vi>)
            n99 = control-ref of="3"() -> (w297:refnum<vi>)
            n100 = control-ref of="4"() -> (w296:refnum<vi>)
            n101 = control-ref of="5"() -> (w295:refnum<vi>)
            n102 = control-ref of="6"() -> (w294:refnum<vi>)
            n103 = control-ref of="7"() -> (w293:refnum<vi>)
            n104 = control-ref of="8"() -> (w288:refnum<vi>)
            n105 = control-ref of="9"() -> (w286:refnum<vi>)
            n106 = control-ref of="10"() -> (w285:refnum<vi>)
            n107 = control-ref of="11"() -> (w284:refnum<vi>)
            n108 = control-ref of="12"() -> (w283:refnum<vi>)
            n109 = control-ref of="13"() -> (w282:refnum<vi>)
            n110 = control-ref of="14"() -> (w281:refnum<vi>)
            n111 = control-ref of="15"() -> (w280:refnum<vi>)
            n112 = Build Array(w299, w298, w297, w296, w295, w294, w293, w288, w286, w285, w284, w283, w282, w281, w280) -> (w287:refnum<vi>[])
            n113 = Bundle By Name(cluster=w307, "Button Ref"=w287) -> (w273:T5)
            n114 = call "eFGV - Start Acquisition.vi"("FGV State"=w267, "Error In"=w269) -> ("Error Out"=w268:errorcluster, "Event Start Acquire"=w266:refnum<user-event>)  [unwired: 7 in, 1 out]
            n115 = call "eFGV - Sequence Data.vi"("States"=w267, "Error In"=w268) -> ("Error Out"=w271:errorcluster, "Event - Sequence Data"=w270:refnum<user-event>)  [unwired: 7 in, 1 out]
            n116 = call "eFGV - Popup.vi"("Action"=w267, "Error In"=w271) -> ("Error Out"=w275:errorcluster, "Event Popup"=w274:refnum<user-event>)  [unwired: 7 in, 1 out]
            n117 = call "eFGV - Logout.vi"("Action"=w267, "Error In"=w275) -> ("Error Out"=w277:errorcluster, "Event Logout"=w276:refnum<user-event>)  [unwired: 7 in, 1 out]
            n118 = call "eFGV - Set Cursor.vi"("FGV State"=w267, "Error In"=w277) -> ("Error Out"=w279:errorcluster, "Event Set Cursor"=w278:refnum<user-event>)  [unwired: 7 in, 1 out]
            n119 = call "eFGV - Update Config.vi"("Action"=w267, "Error In"=w279) -> ("Error Out"=w290:errorcluster, "Event Update Config"=w289:refnum<user-event>)  [unwired: 7 in, 1 out]
            n120 = call "eFGV - Module Run Kill.vi"("Action"=w267, "Error In"=w290) -> ("Error Out"=w292:errorcluster, "Event Module Run Kill"=w291:refnum<user-event>)  [unwired: 7 in, 1 out]
            n121 = Unbundle By Name(w273) -> ("Event Ref"=w265:refnum<event-registration>)
            n122 = call "eFGV - Page Name List.vi"("Action"=w267, "Error In"=w292) -> ("Error Out"=w301:errorcluster, "Event Enable Page"=w300:refnum<user-event>)  [unwired: 7 in, 1 out]
            n123 = call "eFGV - Page Name.vi"("Action"=w267, "Error In"=w301) -> ("Error Out"=w304:errorcluster, "Event Page Name"=w302:refnum<user-event>)  [unwired: 7 in, 1 out]
            n124 = register-events(reference=w265, error in=w304, w302, w300, w291, w289, w278, w276, w274, w270, w266) -> (reference out=w264:refnum<event-registration>, error out=w303:errorcluster)
            n125 = Bundle By Name(cluster=w273, "Event Ref"=w264) -> (w272:T5)
          }
          frame "Init Module" {
            # "Init and run all listed module. If module is running, it will abort  and then run the module."
            n126 = Unbundle By Name(w309) -> ("Config.All HMI Module"=w308:string[])
            n127 = call "FGV - Module Path.vi"("FGV State"=State_-_FGV."Read", "Error In"=w313) -> ("Error Out"=w310:errorcluster, "Path Out"=w311:path)  [unwired: 8 in]
            n128 = call "Gen - SubPanel Page.vi"("State"=T11."Init Module", "Error In"=w310, "Module List"=w308, "Path to Modules Folder"=w311) -> ("Error Out"=w315:errorcluster)  [unwired: 7 in]
          }
          frame "Run Module" {
            # "Init and run all listed module. If module is running, it will abort  and then run the module."
            n129 = Unbundle By Name(w319) -> ("Module.Run Module"=w318:string[])
            n130 = call "Gen - SubPanel Page.vi"("State"=T11."Run Module", "Error In"=w321, "Module List"=w318) -> ("Error Out"=w322:errorcluster)  [unwired: 8 in]
          }
          frame "Kill Module" {
            # "Init and run all listed module. If module is running, it will abort  and then run the module."
            n131 = Unbundle By Name(w326) -> ("Module.Kill Module"=w325:string[])
            n132 = call "Gen - SubPanel Page.vi"("State"=T11."Kill Module", "Error In"=w328, "Module List"=w325) -> ("Error Out"=w329:errorcluster)  [unwired: 8 in]
          }
          frame "Change Page" {
            # "Change to selected page."
            n133 = Unbundle By Name(w353) -> ("Module.Page Module"=w351:string[], "Page Name"=w347:string)
            n134 = Search 1D Array(1D array=w351, element=w347) -> (index of element=w349:i32)  [unwired: 1 in]
            n135 = Less Than 0?(x=w349) -> (x < 0?=w348:bool)
            n136 = case shown="True" w348 {
              tunnel: w350 -> [w360 w370]
              tunnel: [w360 w369] -> w346
              tunnel: w349 -> [w359 _]
              tunnel: [w359 w362] -> w343
              frame False {
              }
              frame True {
                # "#Todo change the 1st page appeared if required"
                # "Page name not match"
                n137 = call "FGV - Login Status.vi"("Action"=enum16{"Read", "Write"}."Read", "Error In"=w370) -> ("Error Out"=w373:errorcluster, "Username Out"=w374:string)  [unwired: 7 in, 1 out]
                n138 = call "User - Get Info.vi"("Info State"=Header_-_User_Management."Access Level", "Error In"=w373, "Username:"=w374) -> ("Error Out"=w369:errorcluster, "Data Out"=w368:string)  [unwired: 7 in]
                n139 = Not Equal?(x="Admin", y=w368) -> (x != y?=w364:bool)
                n140 = Select(t=Header_-_Page."P5 User", s=w364, f=Header_-_Page."P1 Main") -> (s? t:f=w363:T12)
                n141 = Type Cast(type=0 ("index of element"), x=w363) -> (*(type *) &x=w362:i32)
              }
            }
            n142 = Type Cast(type=T1."1" ("Page"), x=w343) -> (*(type *) &x=w344:T1)
            n143 = Unbundle By Name(w353) -> ("Update Button"=w333:bool, "Acquire"=w334:bool, "Page Name"=w332:string)
            n144 = First Call?() -> (First Call?: T/F=w355:bool)
            n145 = property on="Page" class="RadioBtnsControl (strict)"(error in=w346, "Value"=w344) -> (error out=w345:errorcluster)  [unwired: 1 in, 1 out]
            n146 = call "Gen - SubPanel Page.vi"("State"=T11."Change Page", "Module Name"=w332, "Error In"=w345) -> ("Error Out"=w357:errorcluster)  [unwired: 8 in]
            n147 = Select(t=State_-_Main_HMI."Close Splash Screen", s=w355, f=State_-_Main_HMI."Update Button Page") -> (s? t:f=w338:T6)
            n148 = Select(t=State_-_Main_HMI."Update Button Page", s=w333, f=State_-_Main_HMI."Idle") -> (s? t:f=w336:T6)
            n149 = Bundle By Name(cluster=w353, "Update Button"=TRUE) -> (w340:T5)
            n150 = Select(t=w338, s=w334, f=w336) -> (s? t:f=w335:T6)
          }
          frame "Update Button Page" {
            # "Update button depending on current status; login status, access level, discover device, and list of enable page"
            n151 = call "FGV - Login Status.vi"("Action"=enum16{"Read", "Write"}."Read", "Error In"=w387) -> ("Error Out"=w386:errorcluster, "Username Out"=w381:string, "Login?"=w377:bool)  [unwired: 7 in]
            n152 = case shown="True" w377 {
              tunnel: w386 -> [w404 w492]
              tunnel: [w407 w491] -> w380
              tunnel: [w408 T13."Disabled and Grayed Out" ("Disabled")] -> w383
              tunnel: [w406 T13."Disabled and Grayed Out" ("Disabled")] -> w382
              tunnel: w381 -> [w402 _]
              tunnel: [w398 T13."Disabled and Grayed Out" ("Disabled")] -> w376
              tunnel: w375 -> [w393 w487]
              frame True {
                # "If Admin, Acquire button disable"
                # "Login"
                n153 = call "User - Get Info.vi"("Info State"=Header_-_User_Management."Access Level", "Error In"=w404, "Username:"=w402) -> ("Error Out"=w403:errorcluster, "Data Out"=w400:string)  [unwired: 7 in]
                n154 = Unbundle By Name(w393) -> ("Acquire"=w396:bool, "Log"=w395:bool, "Button Ref"=w394:refnum<vi>[])
                n155 = Not Equal?(x=w400, y="Admin") -> (x != y?=w397:bool)
                n156 = for {
                  tunnel: w403 -> [w485]
                  tunnel: [w484] -> w405
                  tunnel: w394 -> [w483] mode=indexing
                  n157 = call "Gen - Button Disable.vi"("State"=enum16{"Enable", "Disable", "Disable & Gray"}."Disable & Gray", "Error In"=w485, "Ref in"=w483) -> ("Error Out"=w484:errorcluster)  [unwired: 8 in]
                }
                n158 = case shown="True" w396 {
                  tunnel: [w412 w472] -> w407
                  tunnel: w405 -> [w417 w473]
                  tunnel: w394 -> [w416 _]
                  tunnel: w395 -> [w414 _]
                  tunnel: [T13."Enabled" ("Disabled") T13."Disabled and Grayed Out" ("Disabled")] -> w406
                  tunnel: [T13."Disabled and Grayed Out" ("Disabled") T13."Enabled" ("Disabled")] -> w398
                  tunnel: w393 -> [w411 w469]
                  frame True {
                    # "Start Acquire"
                    n159 = case shown="True" w414 {
                      tunnel: w416 -> [_ _]
                      tunnel: [w422 w446] -> w412
                      tunnel: w417 -> [w423 w447]
                      tunnel: w411 -> [w424 w448]
                      frame False {
                        # "Stop Log"
                        n160 = Unbundle By Name(w424) -> ("Button Ref"=w419:refnum<vi>[], "Module.Page Module"=w420:string[], "Module.Enable Page"=w421:string[], "Config.Acquire Enable Page"=w418:string[])
                        n161 = for {
                          tunnel: w421 -> [w428]
                          tunnel: w420 -> [w430]
                          tunnel: w419 -> [w429]
                          shift-right: [w431] -> w422
                          shift-left: w423 -> [w432]
                          tunnel: w418 -> [w427] mode=indexing
                          n162 = Equal?(x=w428, y=w427) -> (x = y?=w426:bool[])
                          n163 = Or Array Elements(Boolean array=w426) -> (logical OR=w425:bool)
                          n164 = case shown="True" w425 {
                            tunnel: w432 -> [w433 w441]
                            tunnel: [w433 w440] -> w431
                            tunnel: w430 -> [_ w439]
                            tunnel: w429 -> [_ w438]
                            tunnel: w427 -> [_ w437]
                            frame False {
                            }
                            frame True {
                              n165 = Search 1D Array(1D array=w439, element=w437) -> (index of element=w436:i32)  [unwired: 1 in]
                              n166 = Index Array(array=w438, index=w436) -> (element=w434:refnum<vi>)
                              n167 = call "Gen - Button Disable.vi"("State"=enum16{"Enable", "Disable", "Disable & Gray"}."Enable", "Error In"=w441, "Ref in"=w434) -> ("Error Out"=w440:errorcluster)  [unwired: 8 in]
                            }
                          }
                        }
                      }
                      frame True {
                        # "Start Log"
                        n168 = Unbundle By Name(w448) -> ("Button Ref"=w443:refnum<vi>[], "Module.Page Module"=w444:string[], "Module.Enable Page"=w445:string[], "Config.Log Enable Page"=w442:string[])
                        n169 = for {
                          tunnel: w445 -> [w452]
                          tunnel: w444 -> [w454]
                          tunnel: w443 -> [w453]
                          shift-right: [w455] -> w446
                          shift-left: w447 -> [w456]
                          tunnel: w442 -> [w451] mode=indexing
                          n170 = Equal?(x=w452, y=w451) -> (x = y?=w450:bool[])
                          n171 = Or Array Elements(Boolean array=w450) -> (logical OR=w449:bool)
                          n172 = case shown="True" w449 {
                            tunnel: w456 -> [w457 w465]
                            tunnel: [w457 w464] -> w455
                            tunnel: w454 -> [_ w463]
                            tunnel: w453 -> [_ w462]
                            tunnel: w451 -> [_ w461]
                            frame False {
                            }
                            frame True {
                              n173 = Search 1D Array(1D array=w463, element=w461) -> (index of element=w460:i32)  [unwired: 1 in]
                              n174 = Index Array(array=w462, index=w460) -> (element=w458:refnum<vi>)
                              n175 = call "Gen - Button Disable.vi"("State"=enum16{"Enable", "Disable", "Disable & Gray"}."Enable", "Error In"=w465, "Ref in"=w458) -> ("Error Out"=w464:errorcluster)  [unwired: 8 in]
                            }
                          }
                        }
                      }
                    }
                  }
                  frame False {
                    # "Stop Acquire"
                    n176 = Unbundle By Name(w469) -> ("Button Ref"=w467:refnum<vi>[], "Module.Page Module"=w466:string[], "Module.Enable Page"=w468:string[])
                    n177 = for {
                      tunnel: w466 -> [w481]
                      tunnel: w468 -> [w480] mode=indexing
                      tunnel: w467 -> [w478]
                      shift-right: [w477] -> w472
                      shift-left: w473 -> [w479]
                      n178 = Search 1D Array(1D array=w481, element=w480) -> (index of element=w474:i32)  [unwired: 1 in]
                      n179 = Index Array(array=w478, index=w474) -> (element=w476:refnum<vi>)
                      n180 = call "Gen - Button Disable.vi"("State"=enum16{"Enable", "Disable", "Disable & Gray"}."Enable", "Error In"=w479, "Ref in"=w476) -> ("Error Out"=w477:errorcluster)  [unwired: 8 in]
                    }
                  }
                }
                n181 = Select(t=T13."Enabled" ("Disabled"), s=w397, f=T13."Disabled and Grayed Out" ("Disabled")) -> (s? t:f=w408:T13)
              }
              frame False {
                n182 = Unbundle By Name(w487) -> ("Button Ref"=w486:refnum<vi>[])
                n183 = for {
                  tunnel: w492 -> [w495]
                  tunnel: [w494] -> w491
                  tunnel: w486 -> [w496] mode=indexing
                  n184 = call "Gen - Button Disable.vi"("State"=enum16{"Enable", "Disable", "Disable & Gray"}."Disable & Gray", "Error In"=w495, "Ref in"=w496) -> ("Error Out"=w494:errorcluster)  [unwired: 8 in]
                }
              }
            }
            n185 = property on="Log" class="Bool (strict)"(error in=w380, "DisabledEnum"=w382) -> (error out=w379:errorcluster)  [unwired: 1 in, 1 out]
            n186 = First Call?() -> (First Call?: T/F=w391:bool)
            n187 = property on="Acquire" class="Bool (strict)"(error in=w379, "DisabledEnum"=w383) -> (error out=w378:errorcluster)  [unwired: 1 in, 1 out]
            n188 = Select(t=State_-_Main_HMI."Close Splash Screen", s=w391, f=State_-_Main_HMI."Idle") -> (s? t:f=w388:T6)
            n189 = property on="Logout" class="Bool"(error in=w378, "DisabledEnum"=w376) -> (error out=w384:errorcluster)  [unwired: 1 in, 1 out]
          }
          frame "Close Splash Screen" {
            w503 = u8 0  # Transparency
            w504 = TRUE  # Transparently?
            # "This part done one time only. To visible the main  VI after run all listed module. Then  update the FGV - Load Main Status. This FGV will trigger the Splash Screen to close."
            n190 = Unbundle By Name(w498) -> ("Config.HMI Configuration.HMI State"=w497:T16)
            n191 = control-ref of="This VI"() -> (w505:refnum<vi>)
            n192 = call "Gen - VI Transparency.vi"("State"=w497, "Error In"=w507, "Transparency"=w503, "Transparently?"=w504, "Ref VI"=w505) -> ("Error Out"=w502:errorcluster)  [unwired: 5 in, 1 out]
            n193 = call "FGV - Load Main Status.vi"("Action"=enum16{"Read", "Write"}."Write", "Error In"=w502, "Status in"=TRUE) -> ("Error Out"=w506:errorcluster)  [unwired: 7 in, 1 out]
          }
          frame "Idle" {
            n194 = Unbundle By Name(w513) -> ("T_Out"=w512:i32, "Event Ref"=w511:refnum<event-registration>)
            n195 = event shown="[6] <Event Start Acquire>: User Event" {
              selector: w511 -> [_ _ _ _ _ _ _ _ _ _ _ _ _ _ _ _ _ _ _ _ _ _]
              dyn-events: [_ _ _ _ _ _ _ _ _ _ _ _ _ _ _ _ _ _ _ _ _ _] -> w509
              timeout: w512 -> [_ _ _ _ _ _ _ _ _ _ _ _ _ _ _ _ _ _ _ _ _ _]
              tunnel: [w524 w527 w529 w552 w564 w574 w583 w585 w593 w637 w641 w644 w647 w649 w654 w660 w665 w670 w676 w681 w689 w696] -> w518
              tunnel: w517 -> [w524 w527 w532 w550 w565 w575 w583 w584 w594 w637 w641 w644 w647 w649 w654 w660 w665 w670 w676 w682 w690 w695]
              tunnel: [State_-_Main_HMI."Idle" State_-_Main_HMI."Screenshot" State_-_Main_HMI."Idle" w556 State_-_Main_HMI."Move Button Page" State_-_Main_HMI."Acquire Event" State_-_Main_HMI."Idle" State_-_Main_HMI."Log Event" w601 State_-_Main_HMI."Idle" State_-_Main_HMI."Logout" State_-_Main_HMI."Info" State_-_Main_HMI."Check for Exit" ("f") State_-_Main_HMI."Idle" State_-_Main_HMI."Check for Exit" State_-_Main_HMI."Logout" State_-_Main_HMI."Update Button Page" State_-_Main_HMI."Update Button Page" State_-_Main_HMI."Run Module" State_-_Main_HMI."Change Page" State_-_Main_HMI."Idle" State_-_Main_HMI."Idle"] -> w515
              tunnel: [w522 w525 w531 w555 w562 w576 w581 w590 w600 w635 w639 w643 w648 w651 w655 w657 w662 w667 w673 w683 w692 w698] -> w514
              tunnel: w513 -> [w522 w525 w531 w560 w568 w578 w582 w591 w599 w636 w640 w643 w648 w651 w655 w658 w663 w668 w674 w680 w692 w698]
              event Timeout {
                n196 = event-data() -> ()  [unwired: 1 in, 1 out]
                n197 = Unbundle By Name(w522) -> ("Time"=w520:timestamp)
                n198 = Get Date/Time In Seconds() -> (seconds since 1Jan1904=w521:timestamp)
                n199 = Subtract(x=w521, y=w520) -> (x-y=→"Log Time":dbl)
              }
              event "Screenshot": Value Change {
                n200 = event-data() -> ()  [unwired: 1 in, 6 out]
              }
              event "Alarm Event": Mouse Down {
                n201 = event-data() -> ("Mods.Double Click"=w528:bool)  [unwired: 1 in]
                n202 = case shown="True" w528 {
                  tunnel: w532 -> [w533 w537]
                  tunnel: [w533 w539] -> w529
                  frame False {
                  }
                  frame True {
                    n203 = call "FGV - Module Path.vi"("FGV State"=State_-_FGV."Read", "Error In"=w537) -> ("Error Out"=w536:errorcluster, "Path Out"=w534:path)  [unwired: 8 in]
                    n204 = Build Path(base path=w534, name or relative path="Module - Alarm Event.vi") -> (appended path=w542:path)
                    n205 = Open VI Reference(vi path=w542, error in (no error)=w536) -> (vi reference=w546:refnum<vi>, error out=w548:errorcluster)  [unwired: 4 in]
                    n206 = invoke class="VI" method="FP.Open"(reference=w546, error in=w548, "Activate"=TRUE ("Activate?"), "State"=T16."Standard") -> (reference out=w541:refnum<vi>, error out=w547:errorcluster)  [unwired: 1 in, 3 out]
                    n207 = Close Reference(reference=w541, error in (no error)=w547) -> (error out=w540:errorcluster)
                    n208 = property on="Alarm Event" class="Bool"(error in=w540, "Blinking"=FALSE) -> (error out=w539:errorcluster)  [unwired: 1 in, 1 out]
                  }
                }
              }
              event "Developer": Mouse Down {
                n209 = event-data() -> ("Mods.Double Click"=w554:bool)  [unwired: 1 in]
                n210 = Bundle By Name(cluster=w560, "Page Name"="Module - Developer.vi") -> (w555:T5)
                n211 = call "FGV - Login Status.vi"("Action"=enum16{"Read", "Write"}."Read", "Error In"=w550) -> ("Error Out"=w552:errorcluster, "Login?"=w551:bool)  [unwired: 7 in, 1 out]
                n212 = And(x=w554, y=w551) -> (x .and. y?=w553:bool)
                n213 = Select(t=State_-_Main_HMI."Developer Mode", s=w553, f=State_-_Main_HMI."Idle") -> (s? t:f=w556:T6)
              }
              event "Left", "Right": Value Change {
                n214 = event-data() -> ("CtlRef"=w563:refnum<vi>)  [unwired: 1 in]
                n215 = property class="Bool"(reference=w563, error in=w565) -> (reference out=w567:refnum<vi>, error out=w566:errorcluster, "Label.Text"=w561:string)
                n216 = Close Reference(reference=w567, error in (no error)=w566) -> (error out=w564:errorcluster)
                n217 = Bundle By Name(cluster=w568, "Direction"=w561) -> (w562:T5)
              }
              event "Acquire": Value Change {
                n218 = event-data() -> ("NewVal"=w573:bool)  [unwired: 1 in, 5 out]
                n219 = Select(t="Stop Data Acquisition" ("Tip Strip"), s=w573, f="Start Data Acquisition" ("Tip Strip")) -> (s? t:f=w572:string)
                n220 = Bundle By Name(cluster=w578, "Acquire"=w573) -> (w576:T5)
                n221 = property on="Acquire" class="Bool (strict)"(error in=w575, "TipStrip"=w572) -> (error out=w574:errorcluster)  [unwired: 1 in, 1 out]
              }
              event User Event {
                n222 = event-data() -> ("Start"=w580:bool)  [unwired: 1 in, 4 out]
                n223 = Bundle By Name(cluster=w582, "Acquire"=w580) -> (w581:T5)
              }
              event "Log": Value Change {
                n224 = event-data() -> ("NewVal"=w586:bool)  [unwired: 1 in, 5 out]
                n225 = Select(t="Stop Data Logging" ("Tip Strip"), s=w586, f="Start Data Logging" ("Tip Strip")) -> (s? t:f=w587:string)
                n226 = Bundle By Name(cluster=w591, "Log"=w586) -> (w590:T5)
                n227 = property on="Log" class="Bool (strict)"(error in=w584, "TipStrip"=w587) -> (error out=w585:errorcluster)  [unwired: 1 in, 1 out]
              }
              event "Page": Value Change {
                n228 = event-data() -> ("NewVal"=w598:T1)  [unwired: 1 in]
                n229 = To Long Integer(number=w598) -> (32bit integer=w597:i32)
                n230 = Equal?(x=w597, y=1) -> (x = y?=w595:bool)
                n231 = case shown="True" w595 {
                  tunnel: [State_-_Main_HMI."Change Page" w613] -> w601
                  tunnel: [w608 w614] -> w600
                  tunnel: w599 -> [w607 w615]
                  tunnel: w597 -> [w603 w612]
                  tunnel: w594 -> [w602 w611]
                  tunnel: [w602 w610] -> w593
                  frame False {
                    n232 = Unbundle By Name(w607) -> ("Module.Page Module"=w606:string[])
                    n233 = Index Array(array=w606, index=w603) -> (element=w604:string)
                    n234 = Bundle By Name(cluster=w607, "Page Name"=w604, "Update Button"=FALSE) -> (w608:T5)
                  }
                  frame True {
                    n235 = Unbundle By Name(w615) -> ("Sequence Data"=w617:T4[])
                    n236 = Empty Array?(array=w617) -> (empty?=w616:bool)
                    n237 = case shown="True" w616 {
                      tunnel: w615 -> [w622 w632]
                      tunnel: [w621 w632] -> w614
                      tunnel: [State_-_Main_HMI."Change Page" State_-_Main_HMI."Idle"] -> w613
                      tunnel: w612 -> [w619 _]
                      tunnel: w611 -> [w618 w628]
                      tunnel: [w618 w627] -> w610
                      frame False {
                        n238 = Unbundle By Name(w622) -> ("Module.Page Module"=w625:string[])
                        n239 = Index Array(array=w625, index=w619) -> (element=w623:string)
                        n240 = Bundle By Name(cluster=w622, "Page Name"=w623, "Update Button"=FALSE) -> (w621:T5)
                      }
                      frame True {
                        n241 = property on="Page" class="RadioBtnsControl (strict)"(error in=w628, "Value"=T1."1" ("Page")) -> (error out=w627:errorcluster)  [unwired: 1 in, 1 out]
                        n242 = call "Gen - Popup Single Button (Auto Close).vi"("Message in"="No sequence in sequence list.\nPlease select a Ref. Document.", "Header"="SEQUENCE ERROR") -> ()  [unwired: 8 in, 2 out]
                      }
                    }
                  }
                }
              }
              event User Event {
                n243 = event-data() -> ("Sequence Data"=w634:T4[])  [unwired: 1 in]
                n244 = Bundle By Name(cluster=w636, "Sequence Data"=w634) -> (w635:T5)
              }
              event "Logout": Value Change {
                n245 = event-data() -> ()  [unwired: 1 in, 6 out]
                n246 = Bundle By Name(cluster=w640, "Force Logout?"=FALSE) -> (w639:T5)
              }
              event "Info": Value Change {
                n247 = event-data() -> ()  [unwired: 1 in, 6 out]
              }
              event "Close": Value Change {
                n248 = event-data() -> ()  [unwired: 1 in, 6 out]
              }
              event Panel Resize {
                n249 = event-data() -> ()  [unwired: 1 in, 8 out]
              }
              event Panel Close? {
                n250 = event-data() -> ()  [unwired: 1 in, 4 out]
                n251 = event-data("Discard?"=TRUE) -> ()  [unwired: 1 in, 1 out]
              }
              event User Event {
                # "Get this event when user update thier username. Force logout required."
                n252 = event-data() -> ()  [unwired: 1 in, 5 out]
                n253 = Bundle By Name(cluster=w658, "Force Logout?"=TRUE) -> (w657:T5)
              }
              event User Event {
                n254 = event-data() -> ("Enable Page"=w661:string[])  [unwired: 1 in]
                n255 = Bundle By Name(cluster=w663, "Module.Enable Page"=w661) -> (w662:T5)
              }
              event User Event {
                (unwired) TRUE ("Discover")
                # "Verified the device is discovered. If false, IO Setting is loaded from file."
                n256 = event-data() -> ("New Config"=w666:bool)  [unwired: 1 in]
                n257 = Bundle By Name(cluster=w668, "Discover"=w666) -> (w667:T5)
              }
              event User Event {
                n258 = event-data() -> ("Run Module"=w672:string[], "Kill Module"=w671:string[])  [unwired: 1 in]
                n259 = Bundle By Name(cluster=w674, "Module.Run Module"=w672, "Module.Kill Module"=w671) -> (w673:T5)
              }
              event User Event {
                # "New page name updated"
                n260 = event-data() -> ("Page Name in"=w678:string)  [unwired: 1 in]
                n261 = Unbundle By Name(w680) -> ("Module.Page Module"=w679:string[])
                n262 = Bundle By Name(cluster=w680, "Page Name"=w678) -> (w683:T5)
                n263 = Search 1D Array(1D array=w679, element=w678) -> (index of element=w677:i32)  [unwired: 1 in]
                n264 = disable-structure shown="Enabled" {
                  disable-tunnel: w682 -> [w687 w688]
                  disable-tunnel: [w686 w688] -> w681
                  disable-tunnel: w677 -> [w685 _]
                  frame Disabled {
                    n265 = property on="Page" class="RadioBtnsControl (strict)"(error in=w687, "Value"=w685) -> (error out=w686:errorcluster)  [unwired: 1 in, 1 out]
                  }
                  frame Enabled {
                  }
                }
              }
              event User Event {
                # "Enable & disable background when popup appeared."
                n266 = event-data() -> ("Popup"=w691:bool)  [unwired: 1 in]
                n267 = property on="Disable" class="Bool (strict)"(error in=w690, "Visible"=w691) -> (error out=w689:errorcluster)  [unwired: 1 in, 1 out]
              }
              event User Event {
                # "Set cursor busy and unset busy"
                n268 = event-data() -> ("Cursor Busy In"=w697:bool)  [unwired: 1 in]
                n269 = case shown="False" w697 {
                  tunnel: [w699 w701] -> w696
                  tunnel: w695 -> [w700 w702]
                  frame False {
                    n270 = call <vilib>:"Unset Busy.vi"("error in (no error)"=w700) -> ("error out"=w699:errorcluster)  [unwired: 10 in]
                  }
                  frame True {
                    n271 = call <vilib>:"Set Busy.vi"("error in (no error)"=w702) -> ("error out"=w701:errorcluster)  [unwired: 9 in, 1 out]
                  }
                }
              }
            }
            n272 = Bundle By Name(cluster=w514, "Event Ref"=w509) -> (w510:T5)
          }
          frame "Screenshot" {
            # "Use to screenshot the whole UI and auto save"
            n273 = control-ref of="This VI"() -> (w725:refnum<vi>)
            n274 = invoke class="VI" method="FP.Get Image"(reference=w725, error in=w724) -> (reference out=w726:refnum<vi>, error out=w727:errorcluster, "image data"=w703:T10)  [unwired: 4 in, 3 out]
            n275 = Close Reference(reference=w726, error in (no error)=w727) -> (error out=w713:errorcluster)
            n276 = call "FGV - Data Path.vi"("FGV State"=State_-_FGV."Read", "Error In"=w713) -> ("Error Out"=w712:errorcluster, "Path Out"=w710:path)  [unwired: 8 in]
            n277 = Get Date/Time In Seconds() -> (seconds since 1Jan1904=w722:timestamp)
            n278 = call "FGV - Data Folder.vi"("Action"=enum16{"Read", "Write"}."Read", "Error In"=w712) -> ("Error Out"=w719:errorcluster, "Mode Out"=w721:T24)  [unwired: 8 in]
            n279 = Format Date/Time String(time format string (%c)="%y%m%d %H%M%S ", seconds (now)=w722) -> (date/time string=w717:string)  [unwired: 1 in]
            n280 = Build Path(base path=w710, name or relative path=path "Data/Screenshot") -> (appended path=w709:path)
            n281 = Format Into String(format string="%s", initial string=w717, error in=w719, w721) -> (resulting string=w716:string, error out=w718:errorcluster)
            n282 = Concatenate Strings(w716, ".png" ("string")) -> (w708:string)
            n283 = Build Path(base path=w709, name or relative path=w708) -> (appended path=w706:path)
            n284 = call <vilib>:"Write PNG File.vi"("error in (no error)"=w718, "image data"=w703, "path to PNG file"=w706) -> ("error out"=w705:errorcluster)  [unwired: 7 in, 1 out]
            n285 = call "Screenshot Flash.vi"("Error In"=w705, "Image Data"=w703) -> ("Error Out"=w704:errorcluster)  [unwired: 8 in, 1 out]
          }
          frame "Developer Mode" {
            # "Run developer page as popup."
            n286 = call "Gen - Get Application Kind.vi"("Error In"=w737) -> ("Error Out"=w736:errorcluster)  [unwired: 9 in, 1 out]
            n287 = case shown="\"Run Time System\"" T7."Run Time System" ("Application:Kind") {
              tunnel: [w769 w772 w774] -> w734
              tunnel: [FALSE ("Login?") w771 TRUE ("Login?")] -> w735
              tunnel: w736 -> [w769 w770 w774]
              frame "invalid app kind", Default {
              }
              frame "Run Time System" {
                n288 = call "Login - Developer Mode.vi"("Error In"=w770) -> ("Error Out"=w772:errorcluster, "Login?"=w771:bool)  [unwired: 9 in]
              }
              frame "Development System" {
              }
            }
            n289 = case shown="True" w735 {
              tunnel: w734 -> [w740 w755]
              tunnel: [w740 w751] -> w733
              frame False {
              }
              frame True {
                n290 = call "FGV - Module Path.vi"("FGV State"=State_-_FGV."Read", "Error In"=w755) -> ("Error Out"=w756:errorcluster, "Path Out"=w753:path)  [unwired: 8 in]
                n291 = Build Path(base path=w753, name or relative path="Module - Developer.vi") -> (appended path=w761:path)
                n292 = Open VI Reference(vi path=w761) -> (vi reference=w760:refnum<vi>)  [unwired: 5 in, 1 out]
                n293 = property class="VI"(reference=w760, error in=w756) -> (reference out=w759:refnum<vi>, error out=w758:errorcluster, "Exec.State"=w757:T25)
                n294 = case shown="\"Run top level\", \"Running\"" w757 {
                  tunnel: w758 -> [w763 w767]
                  tunnel: w759 -> [w762 w766]
                  tunnel: [w762 w764] -> w748
                  tunnel: [w763 w765] -> w743
                  frame Default {
                  }
                  frame "Run top level", "Running" {
                    n295 = invoke class="VI" method="Abort VI"(reference=w766, error in=w767) -> (reference out=w764:refnum<vi>, error out=w765:errorcluster)  [unwired: 1 in, 1 out]
                  }
                }
                n296 = invoke class="VI" method="Run VI"(reference=w748, error in=w743, "Wait until done"=FALSE ("Wait Until Done"), "Auto Dispose Ref"=FALSE ("Auto Dispose Reference")) -> (reference out=w747:refnum<vi>, error out=w746:errorcluster)  [unwired: 1 in, 3 out]
                n297 = invoke class="VI" method="FP.Open"(reference=w747, error in=w746, "Activate"=FALSE ("Activate?"), "State"=T16."Standard") -> (reference out=w745:refnum<vi>, error out=w744:errorcluster)  [unwired: 1 in, 3 out]
                n298 = Close Reference(reference=w745, error in (no error)=w744) -> (error out=w751:errorcluster)
              }
            }
          }
          frame "Info" {
            # "Open website link of product."
            n299 = call "aFGV - Read Write Config.vi"("State"=enum16{"Read", "Write", "Delete"}."Read", "Section"=Section."Properties", "Error In"=w779) -> ("Error Out"=w780:errorcluster, "Data out"=w776:string[])  [unwired: 6 in, 1 out]
            n300 = Index Array(array=w776) -> (element=w775:string)  [unwired: 1 in]
            n301 = call-poly <vilib>:"Open URL in Default Browser.vi"("error in (no error)"=w780, "URL"=w775) -> ("error out"=w781:errorcluster)  [unwired: 4 in, 1 out]
          }
          frame "Move Button Page" {
            w798 = i16 80  # Button Size
            n302 = Unbundle By Name(w804) -> ("Page Size (Hidden)"=w786:i32, "Content Area Rect.Left"=w788:i16, "Direction"=w803:string)
            n303 = property on="Page" class="RadioBtnsControl (strict)"(error in=w792) -> (error out=w791:errorcluster, "Controls[]"=w790:refnum<vi>[])  [unwired: 1 in, 1 out]
            n304 = Array Size(array=w790) -> ()  [unwired: 1 out]
            n305 = To Word Integer(number=w786) -> (16bit integer=w789:i16)
            n306 = Multiply(x=w789, y=w798) -> (x*y=w785:i16)
            n307 = property on="Pane 4" class="Pane"(error in=w791) -> (error out=w801:errorcluster, "Origin"=w802:T18)  [unwired: 1 in, 1 out]
            n308 = Add(x=w785, y=w788) -> ()  [unwired: 1 out]
            n309 = case shown="\"Right\", Default" w803 {
              tunnel: [w810 w814] -> w795
              tunnel: w801 -> [w810 w814]
              tunnel: T18 {"Horizontal"=80, "Vertical"=0} ("y") -> [w809 w813]
              tunnel: w802 -> [w808 w812]
              tunnel: [w807 w811] -> w796
              frame "Left" {
                n310 = Subtract(x=w808, y=w809) -> (x-y=w807:T18)
              }
              frame "Right", Default {
                n311 = Add(x=w812, y=w813) -> (x+y=w811:T18)
              }
            }
            n312 = Unbundle By Name(w796) -> ("Horizontal"=w800:i16)
            n313 = In Range and Coerce(upper limit=w785, x=w800, lower limit=i16 0) -> (coerced(x)=w799:i16)  [unwired: 1 out]
            n314 = Bundle By Name(cluster=w796, "Horizontal"=w799) -> (w793:T18)
            n315 = property on="Pane 4" class="Pane"(error in=w795, "Origin"=w793) -> (error out=w794:errorcluster)  [unwired: 1 in, 1 out]
          }
          frame "Acquire Event" {
            # "#Note\nUse for VSys DAQ. Function remain for other project"
            # "Start acquire. Enable/Disable log button depending on license level. Enable/disable related page."
            n316 = Unbundle By Name(w837) -> ("Acquire"=w836:bool)
            n317 = case shown="True" w836 {
              selector: w836 -> [w853 _]
              tunnel: [w850 w861] -> w824
              tunnel: w838 -> [w851 w861]
              tunnel: [w855 w860] -> w831
              tunnel: w837 -> [w856 w860]
              tunnel: [T13."Disabled and Grayed Out" ("Disabled") T13."Enabled" ("Disabled")] -> w832
              tunnel: [T13."Enabled" ("Disabled") T13."Disabled and Grayed Out" ("Disabled")] -> w818
              frame False {
                n318 = local write "Log"(w853) -> ()
                n319 = property on="Log Time" class="DigNum (strict)"(error in=w851, "Visible"=w853) -> (error out=w852:errorcluster)  [unwired: 1 in, 1 out]
                n320 = Bundle By Name(cluster=w856, "T_Out"=-1) -> (w855:T5)
                n321 = call "eFGV - Start Log.vi"("Action"=State_-_eFGV."Write", "Error In"=w852, "Start Log"=w853) -> ("Error Out"=w850:errorcluster)  [unwired: 6 in, 2 out]
              }
              frame True {
                # "Start Acquire"
              }
            }
            n322 = property on="Log" class="Bool (strict)"(error in=w824, "DisabledEnum"=w832) -> (error out=w820:errorcluster)  [unwired: 1 in, 1 out]
            n323 = property on="Logout" class="Bool"(error in=w820, "DisabledEnum"=w818) -> (error out=w819:errorcluster)  [unwired: 1 in, 1 out]
            n324 = Unbundle By Name(w831) -> ("Log"=w830:bool, "Config.Page Module"=w816:string[], "Config.Acquire Enable Page"=w815:string[])
            n325 = property on="Page" class="RadioBtnsControl (strict)"(error in=w819) -> (error out=w834:errorcluster, "Controls[]"=w835:refnum<vi>[])  [unwired: 1 in, 1 out]
            n326 = To Long Integer(number=Header_-_Page."P1 Main") -> (32bit integer=w821:i32)
            n327 = for {
              N: 0 -> [_]
              tunnel: w835 -> [w847]
              tunnel: w818 -> [w843]
              tunnel: w816 -> [w842]
              tunnel: w815 -> [w841] mode=indexing
              tunnel: w834 -> [w846]
              tunnel: [w844] -> w833
              n328 = Search 1D Array(1D array=w842, element=w841) -> (index of element=w840:i32)  [unwired: 1 in]
              n329 = Index Array(array=w847, index=w840) -> (element=w845:refnum<vi>)
              n330 = property class="Ctl"(reference=w845, error in=w846, "DisabledEnum"=w843) -> (error out=w844:errorcluster)  [unwired: 1 out]
            }
            n331 = Index Array(array=w816, index=w821) -> (element=w822:string)
            n332 = Bundle By Name(cluster=w831, "Log"=FALSE, "Page Name"=w822) -> (w826:T5)
            n333 = Select(t=State_-_Main_HMI."Log Event", s=w830, f=State_-_Main_HMI."Change Page") -> (s? t:f=w827:T6)
          }
          frame "Log Event" {
            w870 = -1  # T_Out
            w869 = 500  # T_Out
            # "Event when user start/stop data logging. Update eFGV - Start Log and update logging time."
            n334 = Unbundle By Name(w866) -> ("Log"=w865:bool)
            n335 = call "eFGV - Start Log.vi"("Action"=State_-_eFGV."Write", "Error In"=w867, "Start Log"=w865) -> ("Error Out"=w872:errorcluster)  [unwired: 6 in, 2 out]
            n336 = property on="Log Time" class="DigNum (strict)"(error in=w872, "Visible"=w865, "Value"=0.0 ("Log Time")) -> (error out=w871:errorcluster)  [unwired: 1 in, 1 out]
            n337 = Select(t=w869, s=w865, f=w870) -> (s? t:f=w874:i32)
            n338 = disable-structure shown="Disabled" {
              disable-tunnel: w871 -> [w896 w913]
              disable-tunnel: w865 -> [w892 _]
              disable-tunnel: [w891 w913] -> w862
              frame Disabled {
                n339 = property on="Page" class="RadioBtnsControl (strict)"(error in=w896) -> (error out=w897:errorcluster, "Controls[]"=w898:refnum<vi>[])  [unwired: 1 in, 1 out]
                n340 = Select(t=T13."Disabled and Grayed Out" ("Disabled"), s=w892, f=T13."Enabled") -> (s? t:f=w890:T13)
                n341 = for {
                  N: 0 -> [_]
                  tunnel: w898 -> [w912]
                  tunnel: w890 -> [w909]
                  tunnel: i32[] [4, 5, 6] ("index") -> [w908] mode=indexing
                  shift-right: [w907] -> w889
                  shift-left: w897 -> [w911]
                  n342 = Index Array(array=w912, index=w908) -> (element=w910:refnum<vi>)
                  n343 = property class="Ctl"(reference=w910, error in=w911, "DisabledEnum"=w909) -> (error out=w907:errorcluster)  [unwired: 1 out]
                }
                n344 = call "FGV - Login Status.vi"("Action"=enum16{"Read", "Write"}."Read", "Error In"=w889) -> ("Error Out"=w879:errorcluster, "Username Out"=w882:string)  [unwired: 7 in, 1 out]
                n345 = call "User - Get Info.vi"("Info State"=Header_-_User_Management."Access Page", "Error In"=w879, "Username:"=w882) -> ("Error Out"=w878:errorcluster)  [unwired: 7 in, 1 out]
                n346 = call "Gen - System Config.vi"() -> ("Data Out"=w887:T2)  [unwired: 11 in]
                n347 = Unbundle By Name(w887) -> ("Page Module"=w884:string[], "Default RT Run Module"=w883:string[])
                n348 = property on="Page" class="RadioBtnsControl (strict)"(error in=w878) -> (error out=w885:errorcluster, "Controls[]"=w886:refnum<vi>[])  [unwired: 1 in, 1 out]
                n349 = for {
                  N: 0 -> [_]
                  tunnel: w886 -> [w906]
                  tunnel: w890 -> [w902]
                  tunnel: w884 -> [w901]
                  tunnel: w883 -> [w900] mode=indexing
                  tunnel: w885 -> [w905]
                  tunnel: [w903] -> w891
                  n350 = Search 1D Array(1D array=w901, element=w900) -> (index of element=w899:i32)  [unwired: 1 in]
                  n351 = Index Array(array=w906, index=w899) -> (element=w904:refnum<vi>)
                  n352 = property class="Ctl"(reference=w904, error in=w905, "DisabledEnum"=w902) -> (error out=w903:errorcluster)  [unwired: 1 out]
                }
              }
              frame Enabled {
              }
            }
            n353 = Get Date/Time In Seconds() -> (seconds since 1Jan1904=w873:timestamp)
            n354 = Bundle By Name(cluster=w866, "T_Out"=w874, "Time"=w873) -> (w864:T5)
          }
          frame "Logout" {
            n355 = call "eFGV - Start Acquisition.vi"("FGV State"=State_-_eFGV."Read", "Error In"=w916) -> ("Error Out"=w914:errorcluster, "Start Out"=w915:bool)  [unwired: 7 in, 1 out]
            n356 = case shown="False" w915 {
              tunnel: [w930 State_-_Main_HMI."Idle"] -> w922
              tunnel: [w929 w957] -> w920
              tunnel: w919 -> [w924 w957]
              tunnel: [w928 w952] -> w918
              tunnel: w914 -> [w925 w953]
              frame False {
                n357 = Unbundle By Name(w924) -> ("Force Logout?"=w923:bool)
                n358 = case shown="True" w923 {
                  selector: w923 -> [_ w939]
                  tunnel: [w935 w938] -> w927
                  tunnel: [w933 w939] -> w926
                  tunnel: w925 -> [w931 w938]
                  frame False {
                    n359 = call "Gen - Popup Two Button.vi"("Type"=enum16{"Error", "Info"}."Error", "Error in"=w931, "Button text"=string[] ["YES", "NO"], "Message in"="Are you sure to logout?", "Header"="Logout") -> ("Error out"=w935:errorcluster, "Yes?"=w933:bool)  [unwired: 5 in]
                  }
                  frame True {
                  }
                }
                n360 = case shown="True" w926 {
                  tunnel: [State_-_Main_HMI."Idle" State_-_Main_HMI."Change Page"] -> w930
                  tunnel: [w941 w948] -> w929
                  tunnel: w924 -> [w941 w947]
                  tunnel: w927 -> [w940 w943]
                  tunnel: [w940 w946] -> w928
                  frame False {
                  }
                  frame True {
                    n361 = call "FGV - Login Status.vi"("Action"=enum16{"Read", "Write"}."Write", "Error In"=w943, "Login In"=FALSE) -> ("Error Out"=w946:errorcluster)  [unwired: 6 in, 2 out]
                    n362 = Bundle By Name(cluster=w947, "Page Name"="Module - Login.vi") -> (w948:T5)
                  }
                }
              }
              frame True {
                n363 = call "Gen - Popup Single Button (Auto Close).vi"("Type"=enum16{"Error", "Info"}."Error", "Error in"=w953, "Message in"="Data acquisiton in progress.\n\nPlease stop an acquisition before logout.", "Header"="Exit") -> ("Error out"=w952:errorcluster)  [unwired: 6 in, 1 out]
              }
            }
          }
          frame "Check for Exit" {
            # "Decline exit if Data acquisition in progress."
            n364 = call "eFGV - Start Acquisition.vi"("FGV State"=State_-_eFGV."Read", "Error In"=w963) -> ("Error Out"=w961:errorcluster, "Start Out"=w959:bool)  [unwired: 7 in, 1 out]
            n365 = case shown="False" w959 {
              tunnel: w961 -> [w971 w979]
              tunnel: [w970 w978] -> w960
              tunnel: [w969 FALSE ("Yes?")] -> w958
              frame False {
                n366 = call "Gen - Popup Two Button.vi"("Type"=enum16{"Error", "Info"}."Error", "Error in"=w971, "Message in"="Are you sure to close an application?", "Header"="Exit") -> ("Error out"=w970:errorcluster, "Yes?"=w969:bool)  [unwired: 6 in]
              }
              frame True {
                n367 = call "Gen - Popup Single Button (Auto Close).vi"("Error in"=w979, "Message in"="Data acquisiton in progress.\n\nPlease stop an acquisition before exit.", "Header"="Exit") -> ("Error out"=w978:errorcluster)  [unwired: 7 in, 1 out]
              }
            }
            n368 = Select(t=State_-_Main_HMI."Close", s=w958, f=State_-_Main_HMI."Idle") -> (s? t:f=w966:T6)
          }
          frame "Close" {
            (unwired) TRUE  # Maximum?
            w1001 = u8 100  # Transparency
            w1002 = TRUE  # Transparently?
            n369 = call <vilib>:"Set Busy.vi"("error in (no error)"=w1005) -> ("error out"=w998:errorcluster)  [unwired: 9 in, 1 out]
            n370 = call "eFGV - Stop HMI.vi"("Action"=State_-_eFGV."Write", "Error In"=w998, "Stop HMI? In"=TRUE ("Stop Main? In")) -> ("Error Out"=w997:errorcluster)  [unwired: 6 in, 2 out]
            n371 = call "Gen - SubPanel Page.vi"("State"=T11."Exit", "Error In"=w997) -> ("Error Out"=w996:errorcluster)  [unwired: 9 in]
            n372 = control-ref of="This VI"() -> (w990:refnum<vi>)
            n373 = call "Gen - VI Transparency.vi"("State"=T16."Hidden", "Error In"=w996, "Transparency"=w1001, "Transparently?"=w1002, "Ref VI"=w990) -> ("Error Out"=w984:errorcluster, "Ref VI Out"=w989:refnum<vi>)  [unwired: 5 in]
            n374 = call "Gen - Get Application Kind.vi"("Error In"=w984) -> ("Error Out"=w983:errorcluster, "Application:Kind"=w982:T7)  [unwired: 9 in]
            n375 = Unbundle By Name(w986) -> ("Config.HMI Configuration.HMI State"=w987:T16, "Config.HMI Configuration.Res: Width"=w981:i16, "Config.HMI Configuration.Res: Height"=w980:i16)
            n376 = case shown="\"Development System\"" w982 {
              tunnel: [w1010 w1017] -> w992
              tunnel: [w1009 w1016] -> w991
              tunnel: w989 -> [w1009 w1015]
              tunnel: w987 -> [_ w1014]
              tunnel: w983 -> [w1010 w1013]
              tunnel: w981 -> [_ w1012]
              tunnel: w980 -> [_ w1011]
              frame "Run Time System", Default {
              }
              frame "Development System" {
                n377 = case shown="\"Standard\", Default" w1014 {
                  tunnel: w1013 -> [w1030 w1031]
                  tunnel: [w1028 w1031] -> w1017
                  tunnel: [w1025 w1032] -> w1016
                  tunnel: w1015 -> [w1023 w1032]
                  tunnel: w1012 -> [w1019 _]
                  tunnel: w1011 -> [w1018 _]
                  frame "Standard", Default {
                    (unwired) i16 1356  # Width
                    (unwired) i16 655  # Height
                    # "Enable this when to set the minimum size"
                    n378 = Bundle("Res: Width"=w1019, "Res: Height"=w1018) -> (w1022:cluster{"Res: Width":i16, "Res: Height":i16})  [unwired: 1 in]
                    n379 = Bundle("Res: Height"=w1018, "Res: Width"=w1019) -> (w1020:cluster{"Res: Height":i16, "Res: Width":i16})  [unwired: 1 in]
                    n380 = property class="VI"(reference=w1023, error in=w1030, "Front Panel.Resizeable"=TRUE ("Front Panel Window:Resizable"), "Minimum Panel Size"=w1022, "Front Panel.Resizeable"=FALSE ("Front Panel Window:Resizable")) -> (reference out=w1026:refnum<vi>, error out=w1029:errorcluster)
                    n381 = invoke class="VI" method="FP.Run-Time Position.Centered"(reference=w1026, error in=w1029, "Monitor"=i16 0, "Monitor"=w1020) -> (reference out=w1025:refnum<vi>, error out=w1028:errorcluster)  [unwired: 1 in, 3 out]
                  }
                  frame "Maximized" {
                    # "Max size"
                  }
                }
              }
            }
            n382 = Unbundle By Name(w986) -> ("Event Ref"=w985:refnum<event-registration>)
            n383 = Close Reference(reference=w991, error in (no error)=w992) -> (error out=w993:errorcluster)
            n384 = call "Exit Screen.vi"("Error In"=w993) -> ("Error Out"=w994:errorcluster)  [unwired: 9 in, 1 out]
            n385 = Unregister For Events(event registration refnum=w985, error in=w994) -> (error out=w1006:errorcluster)
            n386 = Wait (ms)(milliseconds to wait=u32 2000) -> ()  [unwired: 1 out]
            n387 = call <vilib>:"Unset Busy.vi"("error in (no error)"=w1006) -> ("error out"=w1004:errorcluster)  [unwired: 10 in]
          }
        }
      }
      frame Error {
        n388 = call <vilib>:"Clear Errors.vi"("error in (no error)"=w1037) -> ("error out"=w1039:errorcluster)  [unwired: 5 in, 1 out]
        n389 = call "Gen - Get Application Kind.vi"("Error In"=w1039) -> ("Error Out"=w1035:errorcluster, "Application:Kind"=w1038:T7)  [unwired: 9 in]
        n390 = Format Into String(error in=w1035, w1034) -> (resulting string=w1033:string)  [unwired: 2 in, 1 out]
        n391 = case shown="\"Development System\"" w1038 {
          tunnel: [w1044 w1049 w1053] -> w1036
          tunnel: w1037 -> [w1044 w1046 w1051]
          tunnel: w1033 -> [_ w1045 _]
          frame "invalid app kind", Default {
          }
          frame "Run Time System" {
            n392 = control-ref of="This VI"() -> (w1047:refnum<vi>)
            n393 = call "eFGV - Generated Error.vi"("eFGV States"=State_-_eFGV."Write", "Error In"=w1046, "State"=w1045, "This VI"=w1047) -> ("Error Out"=w1049:errorcluster)  [unwired: 6 in, 1 out]
          }
          frame "Development System" {
            n394 = call <vilib>:"Simple Error Handler.vi"("error in (no error)"=w1051) -> ("error?"=w1050:bool, "error out"=w1052:errorcluster)  [unwired: 4 in, 3 out]
            n395 = case shown="False" w1050 {
              tunnel: [w1054 w1056] -> w1053
              tunnel: w1052 -> [w1054 w1055]
              frame False {
              }
              frame True {
                n396 = call <vilib>:"Clear Errors.vi"("error in (no error)"=w1055) -> ("error out"=w1056:errorcluster)  [unwired: 5 in, 1 out]
              }
            }
          }
        }
        n397 = Wait (ms)(milliseconds to wait=u32 3000) -> ()  [unwired: 1 out]
      }
    }
    n398 = Wait (ms)(milliseconds to wait=u32 100) -> ()  [unwired: 1 out]
  }
  n399 = disable-structure shown="Disabled" {
    frame Disabled {
      n400 = case shown="True" {
        selector: _ -> [_ _]
        tunnel: [w1066 w1100] -> _
        tunnel: _ -> [w1067 w1101]
        tunnel: _ -> [w1061 _]
        tunnel: _ -> [w1062 w1096]
        tunnel: _ -> [w1065 w1099]
        tunnel: _ -> [w1063 w1097]
        tunnel: [T13."Enabled" ("Disabled") T13."Disabled and Grayed Out" ("Disabled")] -> _
        tunnel: [T13."Disabled and Grayed Out" ("Disabled") T13."Enabled" ("Disabled")] -> _
        tunnel: _ -> [w1059 w1094]
        tunnel: _ -> [w1058 w1093]
        tunnel: _ -> [w1057 w1092]
        frame True {
          # "Start Acquire"
          n401 = Unbundle By Name(w1057) -> ()  [unwired: 1 out]
          n402 = for {
            tunnel: w1062 -> [w1078]
            tunnel: w1061 -> [w1077] mode=indexing
            tunnel: w1065 -> [w1075]
            tunnel: w1063 -> [w1074]
            shift-right: [w1072] -> w1066
            shift-left: w1067 -> [w1076]
            tunnel: w1059 -> [w1069] mode=indexing
            tunnel: w1058 -> [w1068] mode=indexing
            n403 = case shown="True" w1074 {
              tunnel: w1075 -> [w1084 w1090]
              tunnel: w1078 -> [w1083 w1089]
              tunnel: w1077 -> [_ _]
              tunnel: [w1081 w1087] -> w1071
              tunnel: [w1080 w1086] -> w1073
              tunnel: w1076 -> [w1080 w1086]
              tunnel: w1069 -> [w1079 _]
              tunnel: w1068 -> [_ w1085]
              frame False {
                # "Stop Log"
                n404 = Search 1D Array(1D array=w1083, element=w1079) -> (index of element=w1082:i32)  [unwired: 1 in]
                n405 = Index Array(array=w1084, index=w1082) -> (element=w1081)
              }
              frame True {
                # "Start Log"
                n406 = Search 1D Array(1D array=w1089, element=w1085) -> (index of element=w1088:i32)  [unwired: 1 in]
                n407 = Index Array(array=w1090, index=w1088) -> (element=w1087)
              }
            }
            n408 = call "Gen - Button Disable.vi"("State"=enum16{"Enable", "Disable", "Disable & Gray"}."Enable", "Error In"=w1073, "Ref in"=w1071) -> ("Error Out"=w1072:errorcluster)  [unwired: 8 in]
          }
        }
        frame False {
          # "Stop Acquire"
          n409 = Unbundle By Name(w1092) -> ("Module.Enable Page"=w1091)
          n410 = for {
            tunnel: w1096 -> [w1112]
            tunnel: w1091 -> [w1111]
            tunnel: w1099 -> [w1109]
            tunnel: w1097 -> [w1108]
            shift-right: [w1106] -> w1100
            shift-left: w1101 -> [w1110]
            tunnel: w1094 -> [w1103] mode=indexing
            tunnel: w1093 -> [w1102] mode=indexing
            n411 = case shown="True" w1108 {
              tunnel: w1109 -> [w1118 w1124]
              tunnel: w1112 -> [w1117 w1123]
              tunnel: w1111 -> [w1116 w1122]
              tunnel: [w1114 w1120] -> w1105
              tunnel: [w1113 w1119] -> w1107
              tunnel: w1110 -> [w1113 w1119]
              tunnel: w1103 -> [_ _]
              tunnel: w1102 -> [_ _]
              frame False {
                # "Stop Log"
                n412 = Search 1D Array(1D array=w1117, element=w1116) -> (index of element=w1115:i32)  [unwired: 1 in]
                n413 = Index Array(array=w1118, index=w1115) -> (element=w1114)
              }
              frame True {
                # "Start Log"
                n414 = Search 1D Array(1D array=w1123, element=w1122) -> (index of element=w1121:i32)  [unwired: 1 in]
                n415 = Index Array(array=w1124, index=w1121) -> (element=w1120)
              }
            }
            n416 = call "Gen - Button Disable.vi"("State"=enum16{"Enable", "Disable", "Disable & Gray"}."Enable", "Error In"=w1107, "Ref in"=w1105) -> ("Error Out"=w1106:errorcluster)  [unwired: 8 in]
          }
        }
      }
    }
    frame Enabled {
    }
  }
  n417 = call "Main - Init Close Variable.vi"("State"=enum16{"Init", "Close"}."Close", "Error In"=w18) -> ("Error Out"=w17:errorcluster)  [unwired: 9 in]
  n418 = control-ref of="This VI"() -> (w15:refnum<vi>)
  n419 = call "Gen - Close VI.vi"("Error In"=w17, "Ref VI"=w15) -> ("Error Out"=→"Error out":errorcluster)  [unwired: 9 in]
